vi "ME_acquire_15_DeltaForce_Daq_steppingMode.vi"() -> ()   [LabVIEW 2015]
doc: "Use this template to build a producer/consumer design pattern. Use this template when you need to execute a process, such as data analysis, when a data source, such as a triggered acquisition, produces data at an uneven rate and you need to execute the process when the data becomes available."
uses:
  oxford_driver/Oxford Drivers/BUSGEN.LLB/OxfordAddress.ctl
  <vilib>/express/express arith-compare/Formula/XNode/ExpressFormulaBlockNode.xnode
  Mode.ctl
  <vilib>/Utility/file.llb/Write Delimited Spreadsheet (DBL).vi
  <vilib>/Analysis/NI_AALBase.lvlib
  <vilib>/Analysis/baseanly.llb/Mean (DBL).vi
  <vilib>/DAQmx/configure/timing.llb/DAQmx Timing (Sample Clock).vi
  <vilib>/DAQmx/create/channels.llb/DAQmx Create Channel (AI-Voltage-Basic).vi
  <vilib>/DAQmx/read.llb/DAQmx Read (Analog 1D DBL 1Chan NSamp).vi
panel:
  out "remaining elements 2":T1(array[cluster])
  out "Actual mean":dbl format="%0.6f"
  in  "Averaged dt":dbl[][](array[numeric])
  in  "Averaged P(B)":dbl[][](array[numeric])
  out "LockInR":dbl
  out "deltaUaux":dbl
  out "Actual Voltage (V)":dbl caption="Actual AuxV" step=0.1
  in  "Stop":bool
  out "SaveSweep":bool=TRUE
  out "Measurement File_dn":path
  out "Measurement File_up":path
  out "Measurement File_average":path
  out "Actual Polarization":dbl
  in  "Reset IB?":bool
  in  "First?":bool
  in  "Save Period":dbl=1.0
  out "Averaged I(B)":dbl[][](array[numeric])
  out "P(uC/mm^2)":dbl[](array[numeric])
  in  "Sweep":bool
  out "Offset array":dbl[](array[numeric])
  in  "stop 2":bool
  in  "dB":dbl=0.005
  in  "Dwell Time (ms)":u32=1
  out "appended array":dbl[][](array[numeric])
  out "Actual B Field (T)":dbl
  out "Actual Temperature (K)":dbl
  out "Actual Current (pA)":dbl
  in  "Tab Control":T2(tab)
  in  "Max temperature (K)":dbl=20.0
  in  "Min Temperature (K)":dbl=4.5
  out "P(T)":cluster{"yi":dbl[], dbl[]}(graph)
  out "I(T)":cluster{dbl[], dbl[]}(graph)
  in  "Set temperature (K)":dbl=4.5
  in  "Temp Ramping Rate (K/min)":dbl=10.0
  in  "Heater Range":enum16{"Off", "Low", "Medium", "High"}(ring)
  in  "Heater On/Off":bool
  out "Setpoint Temperature (K)":dbl
  in  "StepField":bool
  out "I(B) 3":cluster{dbl[], dbl[]}[](graph)
  out "I(B) /Averaged/":cluster{"B array":dbl[], dbl[]}[](graph)
  out "P(B) /Averaged/":cluster{"B array":dbl[], dbl[]}[](graph)
  out "P(B)":cluster{"yi":dbl[], dbl[]}(graph)
  in  "Set Field (T)":dbl
  in  "Go to Set":bool
  in  "Sweep Rate (T/min)":dbl=2.0 format="%.6f"
  in  "Field To Zero":bool
  out "Target Field":dbl
  in  "Min Field (T)":dbl
  in  "Max Field (T)":dbl=0.15
  in  "Threshold B (T)":dbl
  out "Up/Down":bool
  in  "Dwell Time (s)":dbl=0.1
  in  "Max count array":i32[](array[numeric])=[2, 1, 0, 0, 0, 9, 10, 11, 12]
  in  "secs to wait":dbl=180.0
  out "Wait (s)":dbl
  in  "Directory":string
  out "Finished":bool=TRUE
  out "Step Rate":bool
  out "New":bool=TRUE
  in  "Temperature Array":dbl[](array[numeric])=[4.5, 5.0, 6.0, 7.0, 8.0, 9.0, 10.0, 11.0, 12.0]
  in  "Sweep Rate Array":dbl[](array[numeric])=[2.0, 1.0, 0.5, 0.1, 0.05, 9.0, 10.0, 11.0, 12.0]
  in  "Record ALL":bool
  in  "Max Countl":i32
  out "i":i32
  out "j":i32
  out "Step Temp":bool
  in  "FileName":string
  in  "Measure Noise":bool
  in  "Cycles":i32
  in  "maximum value":dbl=10.0 format="%0.2f"
  in  "minimum value":dbl=-10.0 format="%0.2f"
  in  "physical channels":tag="Dev1/ai1"
  out "PSD (pA/Hz^1/2) Peaks Removed":cluster{"f0":dbl, "df":dbl, "magnitude":dbl[]}(graph)
  out "PSD (pA/Hz^1/2)":cluster{"f0":dbl, "df":dbl, "magnitude":dbl[]}(graph)
  out "Current (pA) Filtered":waveform(dbl)(graph)
  out "Current (pA)":dbl[](graph)
  in  "Samples per channel":i32=1000
  in  "Rate":dbl=1000.0 format="%0.2f"
  in  "Cut-Off Frequency":dbl=100.0 caption="Lower Cut-Off"
  in  "Filter On":bool
  in  "First offset?":bool
  in  "Lock_in_Amplifier":refnum<visa-resource-name>="GPIB0::5::INSTR"
  out "Dc offset":dbl
  in  "Calibrate":bool
  in  "IV converter":refnum<visa-resource-name>="GPIB0::20::INSTR"
  in  "Magnetic Field":refnum<visa-resource-name>="GPIB0::21::INSTR"
  out "Time Lag":dbl=0.0500025749206543
  in  "Lake Shore":refnum<visa-resource-name>="GPIB0::11::INSTR"
  in  "Temp Refresh (s)":dbl=0.1
  in  "Sampling rate (Hz)":dbl=10.0
  in  "Gain (V/A)":dbl=1000000000.0
  in  "Sample area (mm^2)":dbl=3.9
  out "B_V":cluster{dbl[], "Best Linear Fit":dbl[]}[](graph)=[{[-0.00854253601, 0.00626134724, 0.0219834428, 0.0379117736, 0.0535871506, 0.0694316728, 0.0851615152, 0.100816481, 0.116478038, 0.132148461, 0.147876163, 0.16341701, 0.178976744, 0.194563632, 0.210251739, 0.225738944, 0.241298253, 0.256806034, 0.272344374, 0.287933477, 0.303494709, 0.318997125, 0.334591297, 0.350146681, 0.365618053, 0.380940961, 0.39666457, 0.412213675, 0.427724671, 0.443221444, 0.458760641, 0.474360042, 0.489915118, 0.505330598, 0.520967119, 0.536347531, 0.551813711, 0.567441155, 0.582995861, 0.598507522, 0.614041988, 0.629563151, 0.645106262, 0.660611914, 0.676136149, 0.691553948, 0.7071244, 0.72262999, 0.738171137, 0.753700392, 0.76919513, 0.784778028, 0.800215944, 0.8156961, 0.831325434, 0.846852183, 0.862326812, 0.877819169, 0.893312568, 0.90888536, 0.924354789], "Best Linear Fit"=[0.0, 0.005, 0.01, 0.015, 0.02, 0.025, 0.03, 0.035, 0.04, 0.045, 0.05, 0.055, 0.06, 0.065, 0.07, 0.075, 0.08, 0.085, 0.09, 0.095, 0.1, 0.105, 0.11, 0.115, 0.12, 0.125, 0.13, 0.135, 0.14, 0.145, 0.15, 0.155, 0.16, 0.165, 0.17, 0.175, 0.18, 0.185, 0.19, 0.195, 0.2, 0.205, 0.21, 0.215, 0.22, 0.225, 0.23, 0.235, 0.24, 0.245, 0.25, 0.255, 0.26, 0.265, 0.27, 0.275, 0.28, 0.285, 0.29, 0.295, 0.3]}, {[-0.00854253601, 0.00626134724, 0.0219834428, 0.0379117736, 0.0535871506, 0.0694316728, 0.0851615152, 0.100816481, 0.116478038, 0.132148461, 0.147876163, 0.16341701, 0.178976744, 0.194563632, 0.210251739, 0.225738944, 0.241298253, 0.256806034, 0.272344374, 0.287933477, 0.303494709, 0.318997125, 0.334591297, 0.350146681, 0.365618053, 0.380940961, 0.39666457, 0.412213675, 0.427724671, 0.443221444, 0.458760641, 0.474360042, 0.489915118, 0.505330598, 0.520967119, 0.536347531, 0.551813711, 0.567441155, 0.582995861, 0.598507522, 0.614041988, 0.629563151, 0.645106262, 0.660611914, 0.676136149, 0.691553948, 0.7071244, 0.72262999, 0.738171137, 0.753700392, 0.76919513, 0.784778028, 0.800215944, 0.8156961, 0.831325434, 0.846852183, 0.862326812, 0.877819169, 0.893312568, 0.90888536, 0.924354789], "Best Linear Fit"=[-0.00022554388023060128, 0.004536267537808887, 0.009593430775915074, 0.014716931562355689, 0.01975906732634002, 0.024855610270593523, 0.029915265354287977, 0.03495083565949541, 0.03998852608757118, 0.045029068349812316, 0.05008803495326229, 0.055086897848955874, 0.060091835929837946, 0.06510550835596321, 0.07015173884687344, 0.07513334727738563, 0.08013814865293042, 0.08512637555172443, 0.0901244320467579, 0.09513881694893507, 0.10014423687592358, 0.10513073807087174, 0.11014675346564809, 0.1151502923271957, 0.12012680792099008, 0.1250555686413888, 0.1301132186920259, 0.13511473785283767, 0.14010399888730068, 0.14508868495702945, 0.1500870171143548, 0.15510471446726903, 0.16010815425765457, 0.16506669165212906, 0.17009632901003072, 0.1750435864450521, 0.18001843198211442, 0.1850451496356715, 0.19004847041199868, 0.1950379453501071, 0.20003475573578386, 0.20502728708357412, 0.21002687821664084, 0.21501442030211, 0.220007939788244, 0.2249672231113706, 0.22997560874002893, 0.23496313088260184, 0.23996209027618054, 0.24495722449359253, 0.24994125598600042, 0.2549536449902534, 0.25991939913989753, 0.2648987401917687, 0.26992606578200207, 0.2749203939204135, 0.2798979571595809, 0.2848812227804405, 0.2898648235706211, 0.2948739618827834, 0.2998498524919418]}]
  out "V_I":cluster{dbl[], "Best Linear Fit":dbl[]}[](graph)=[{[0.0, 0.035, 0.069, 0.104, 0.138, 0.173, 0.208, 0.242, 0.277, 0.311, 0.346, 0.38, 0.415, 0.45, 0.484, 0.519, 0.553, 0.588, 0.623, 0.657, 0.692, 0.726, 0.761, 0.796, 0.83, 0.865, 0.899, 0.934, 0.969, 1.003, 1.038, 1.072, 1.107, 1.141, 1.176, 1.211, 1.245, 1.28, 1.314, 1.349, 1.384, 1.418, 1.453, 1.487, 1.522, 1.557, 1.591, 1.626, 1.66, 1.695, 1.73, 1.764, 1.799, 1.833, 1.868, 1.902, 1.937, 1.972, 2.006, 2.041, 2.075], "Best Linear Fit"=[-0.00854253601, 0.00626134724, 0.0219834428, 0.0379117736, 0.0535871506, 0.0694316728, 0.0851615152, 0.100816481, 0.116478038, 0.132148461, 0.147876163, 0.16341701, 0.178976744, 0.194563632, 0.210251739, 0.225738944, 0.241298253, 0.256806034, 0.272344374, 0.287933477, 0.303494709, 0.318997125, 0.334591297, 0.350146681, 0.365618053, 0.380940961, 0.39666457, 0.412213675, 0.427724671, 0.443221444, 0.458760641, 0.474360042, 0.489915118, 0.505330598, 0.520967119, 0.536347531, 0.551813711, 0.567441155, 0.582995861, 0.598507522, 0.614041988, 0.629563151, 0.645106262, 0.660611914, 0.676136149, 0.691553948, 0.7071244, 0.72262999, 0.738171137, 0.753700392, 0.76919513, 0.784778028, 0.800215944, 0.8156961, 0.831325434, 0.846852183, 0.862326812, 0.877819169, 0.893312568, 0.90888536, 0.924354789]}, {[0.0, 0.035, 0.069, 0.104, 0.138, 0.173, 0.208, 0.242, 0.277, 0.311, 0.346, 0.38, 0.415, 0.45, 0.484, 0.519, 0.553, 0.588, 0.623, 0.657, 0.692, 0.726, 0.761, 0.796, 0.83, 0.865, 0.899, 0.934, 0.969, 1.003, 1.038, 1.072, 1.107, 1.141, 1.176, 1.211, 1.245, 1.28, 1.314, 1.349, 1.384, 1.418, 1.453, 1.487, 1.522, 1.557, 1.591, 1.626, 1.66, 1.695, 1.73, 1.764, 1.799, 1.833, 1.868, 1.902, 1.937, 1.972, 2.006, 2.041, 2.075], "Best Linear Fit"=[-0.007846580254753975, 0.007882153481927697, 0.02316149482613275, 0.03889022856281441, 0.054169569907019474, 0.06989830364370113, 0.08562703738038281, 0.10090637872458785, 0.11663511246126955, 0.1319144538054746, 0.14764318754215625, 0.1629225288863613, 0.17865126262304296, 0.19437999635972467, 0.2096593377039297, 0.22538807144061138, 0.24066741278481643, 0.25639614652149806, 0.27212488025817977, 0.2874042216023848, 0.3031329553390665, 0.31841229668327153, 0.3341410304199532, 0.3498697641566349, 0.3651491055008399, 0.3808778392375216, 0.39615718058172666, 0.4118859143184083, 0.42761464805509, 0.442893989399295, 0.45862272313597674, 0.4739020644801818, 0.48963079821686345, 0.5049101395610684, 0.5206388732977502, 0.5363676070344319, 0.5516469483786369, 0.5673756821153185, 0.5826550234595236, 0.5983837571962053, 0.6141124909328869, 0.629391832277092, 0.6451205660137737, 0.6603999073579787, 0.6761286410946604, 0.691857374831342, 0.7071367161755471, 0.7228654499122288, 0.7381447912564338, 0.7538735249931156, 0.7696022587297972, 0.7848816000740022, 0.8006103338106839, 0.815889675154889, 0.8316184088915707, 0.8468977502357756, 0.8626264839724573, 0.878355217709139, 0.893634559053344, 0.9093632927900257, 0.9246426341342309]}]
  out "B0 (T)":dbl=0.0025222449819540214
  out "B/V (T/V)":dbl=0.321659617116981
  out "I0 (A)":dbl=-0.007846580254753975
  out "V/I (Ohm)":dbl=0.44939239247661916
  in  "Offset?":bool
  in  "Magnet":bool
  in  "Ramp":bool=TRUE
  in  "DaQ":bool
  in  "Moving average":i8=10
  in  "Sample Rate":dbl=1000.0
  in  "Number of Samples":i32=100
  in  "Physical Channel":tag="kartya/ai0"
  in  "Min Voltage":dbl=-5.0
  in  "Max Voltage":dbl=5.0
  in  "Terminal Configuration":i32(ring)=-1 items=["default"=-1, "RSE"=10083, "NRSE"=10078, "Differential"=10106, "Pseudodifferential"=12529]
  in  "Count":i32=100
  in  "Temp/Magnetic Field":bool
  out "index":i8
  out "Read?":bool
  out "Magnetic Field (T)":dbl[](array[numeric])
  out "Reset":bool
  out "Measured Current (pA)":dbl[](array[numeric])
  out "Elapsed Time (s)":dbl[](array[numeric])
  out "Start time":timestamp
  in  "Enum":T3=enum."Process"
  out "B array":dbl[](array[numeric])
  in  "dB (T)":dbl=0.0025
  in  "Counter":i8
  out "L magnet (H)":dbl
  out "R magnet (mOhm)":dbl
  out "Actual Current (R0)":dbl
  out "Actual Field (T)":dbl
  out "Temperature array":dbl[](array[numeric])
  in  "New Measurement File":bool
  out "Measurement File":path
  out "refnum out":refnum<file>
  in  "Measuring":bool
  in  "Measure /Pause":bool
  in  "stop":bool
  # "DeltaForce"
  # "Discrete"
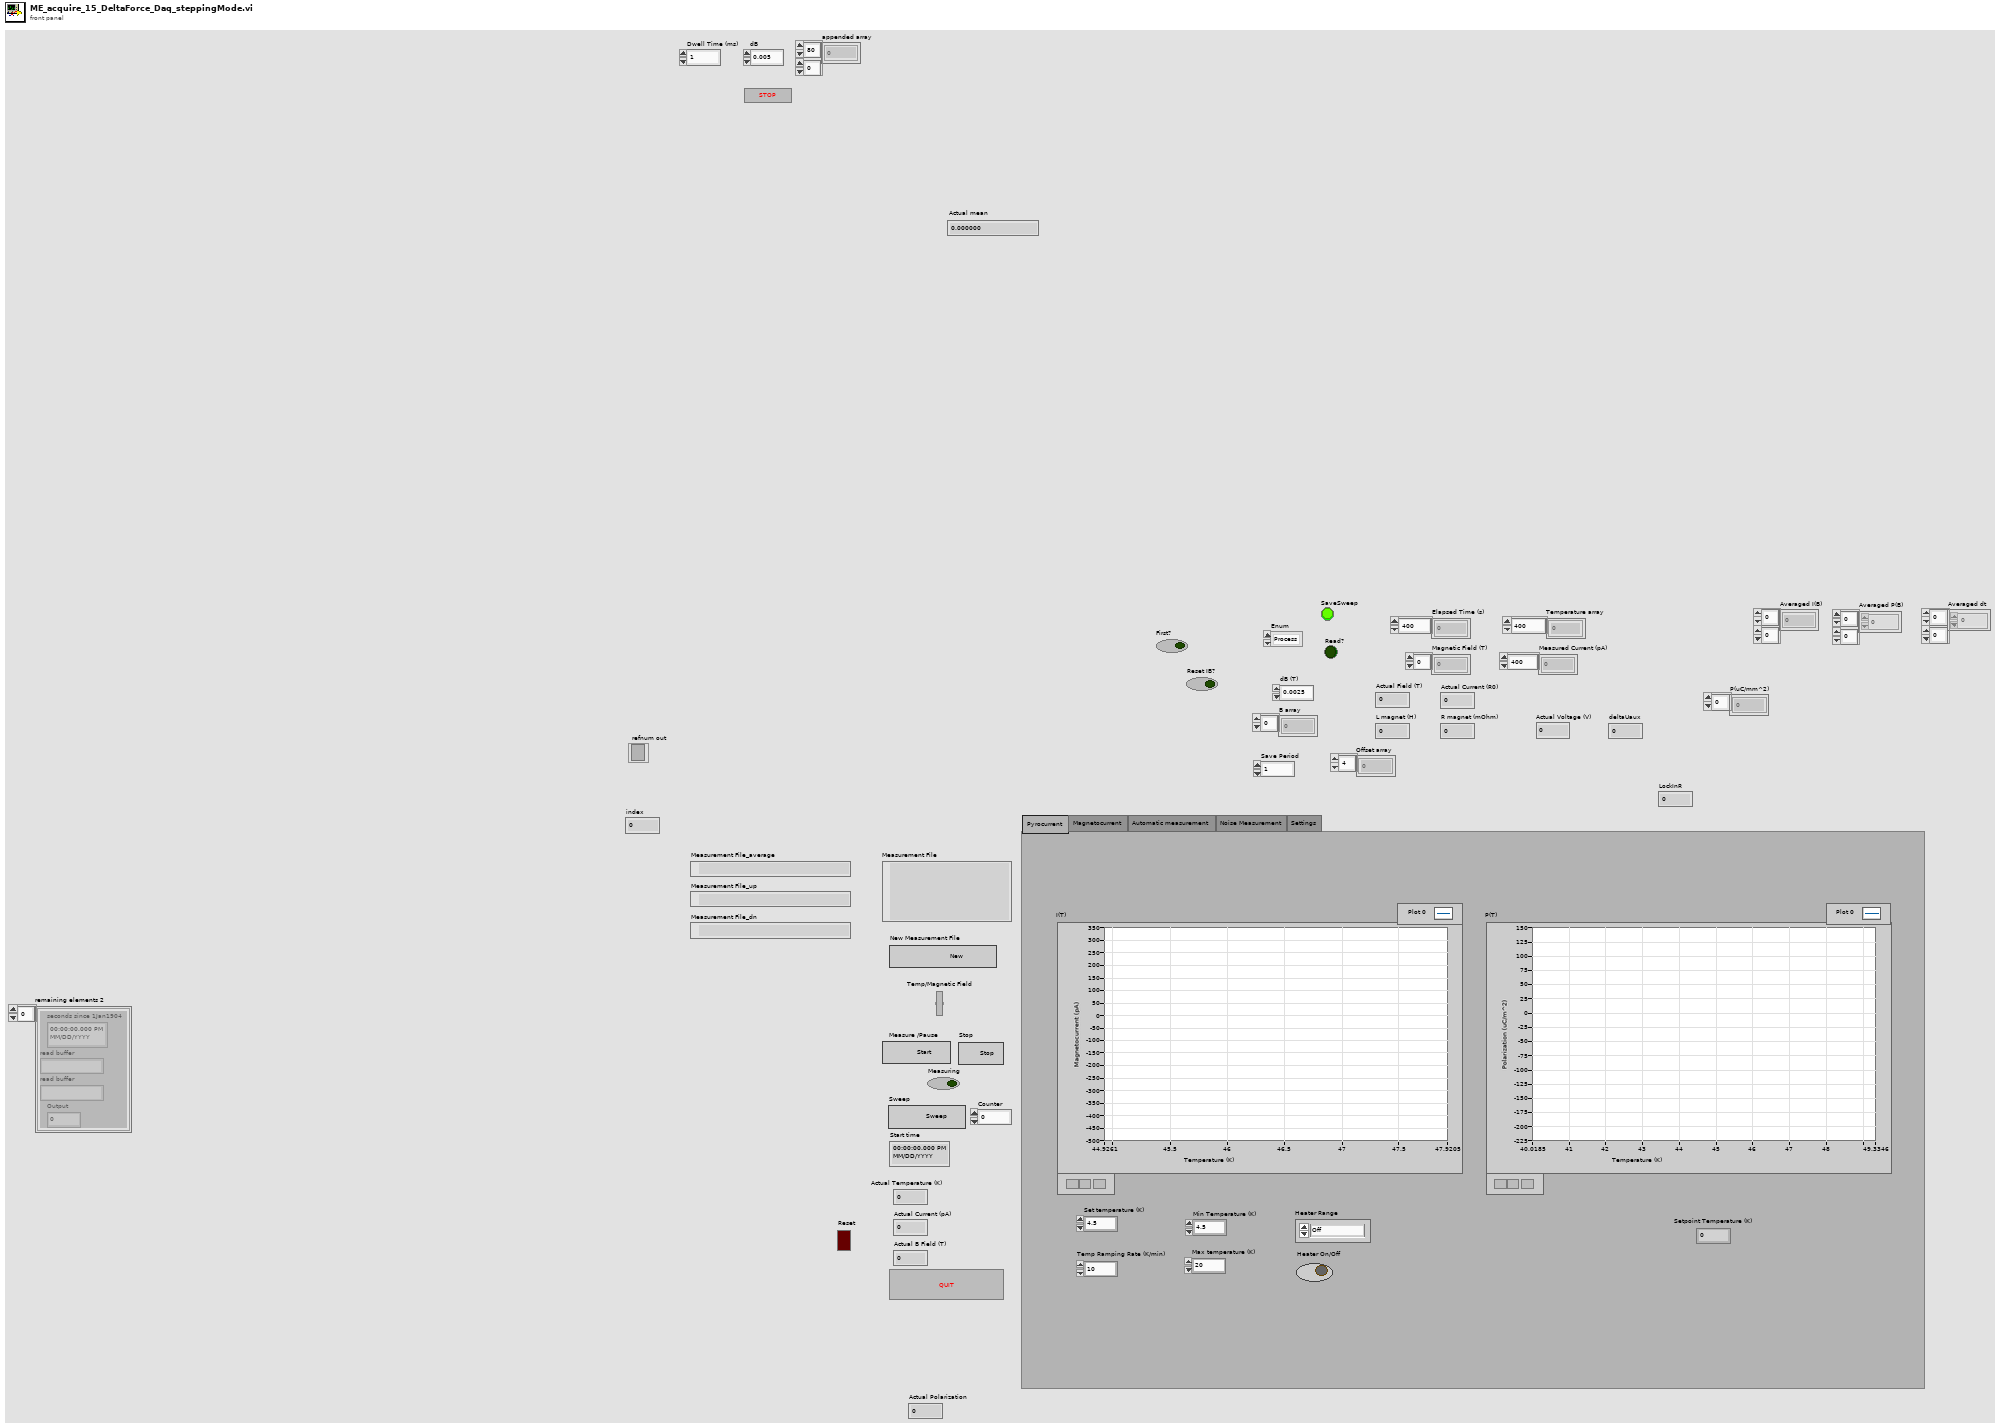
[diagram p1: front panel]
types:
  T1 = cluster{"seconds since 1Jan1904":timestamp, "read buffer":string, "read buffer":string, "Output":dbl}[]
  T2 = enum32{"Pyrocurrent", "Magnetocurrent", "Automatic measurement", "Noise Measurement", "Settings"}
  T3 = typedef "Mode.ctl" = enum16{"Offset", "Process", "Sweep", "StepOxford", "StepDelta", "Plot", "Save", "New", "Return", ""}
  T4 = cluster{"seconds since 1Jan1904":timestamp, "read buffer":string, "read buffer":string, "Output":dbl}
  T5 = enum16{"open", "replace", "create", "open or create", "replace or create", "replace or create with confirmation"}
  T6 = typedef "OxfordAddress.ctl" = cluster{"Com Port":i32, "ISOBUS Address":i32, "GPIB Address":i16, "Communication":enum16{"RS232", "ISOBUS", "GPIB", "Gateway"}}
  T7 = cluster{"B array":dbl[], "Averaged P(B) Out":dbl[]}
  T8 = cluster{"B array":dbl[], "BaselineSubtracted I(B)":dbl[]}
  T9 = cluster{"B array":dbl[], "Averaged P(B) Out":dbl[]}[]
  T10 = cluster{"B array":dbl[], "BaselineSubtracted I(B)":dbl[]}[]
  T11 = cluster{"I array out (A)":dbl[], "V array out (V)":dbl[]}
  T12 = cluster{"I array out (A)":dbl[], "Best Linear Fit":dbl[]}
  T13 = cluster{"V array out (V)":dbl[], "B array Out":dbl[]}
  T14 = cluster{"V array out (V)":dbl[], "Best Linear Fit 2":dbl[]}
  T15 = cluster{"I array out (A)":dbl[], "Best Linear Fit":dbl[]}[]
  T16 = cluster{"V array out (V)":dbl[], "Best Linear Fit 2":dbl[]}[]
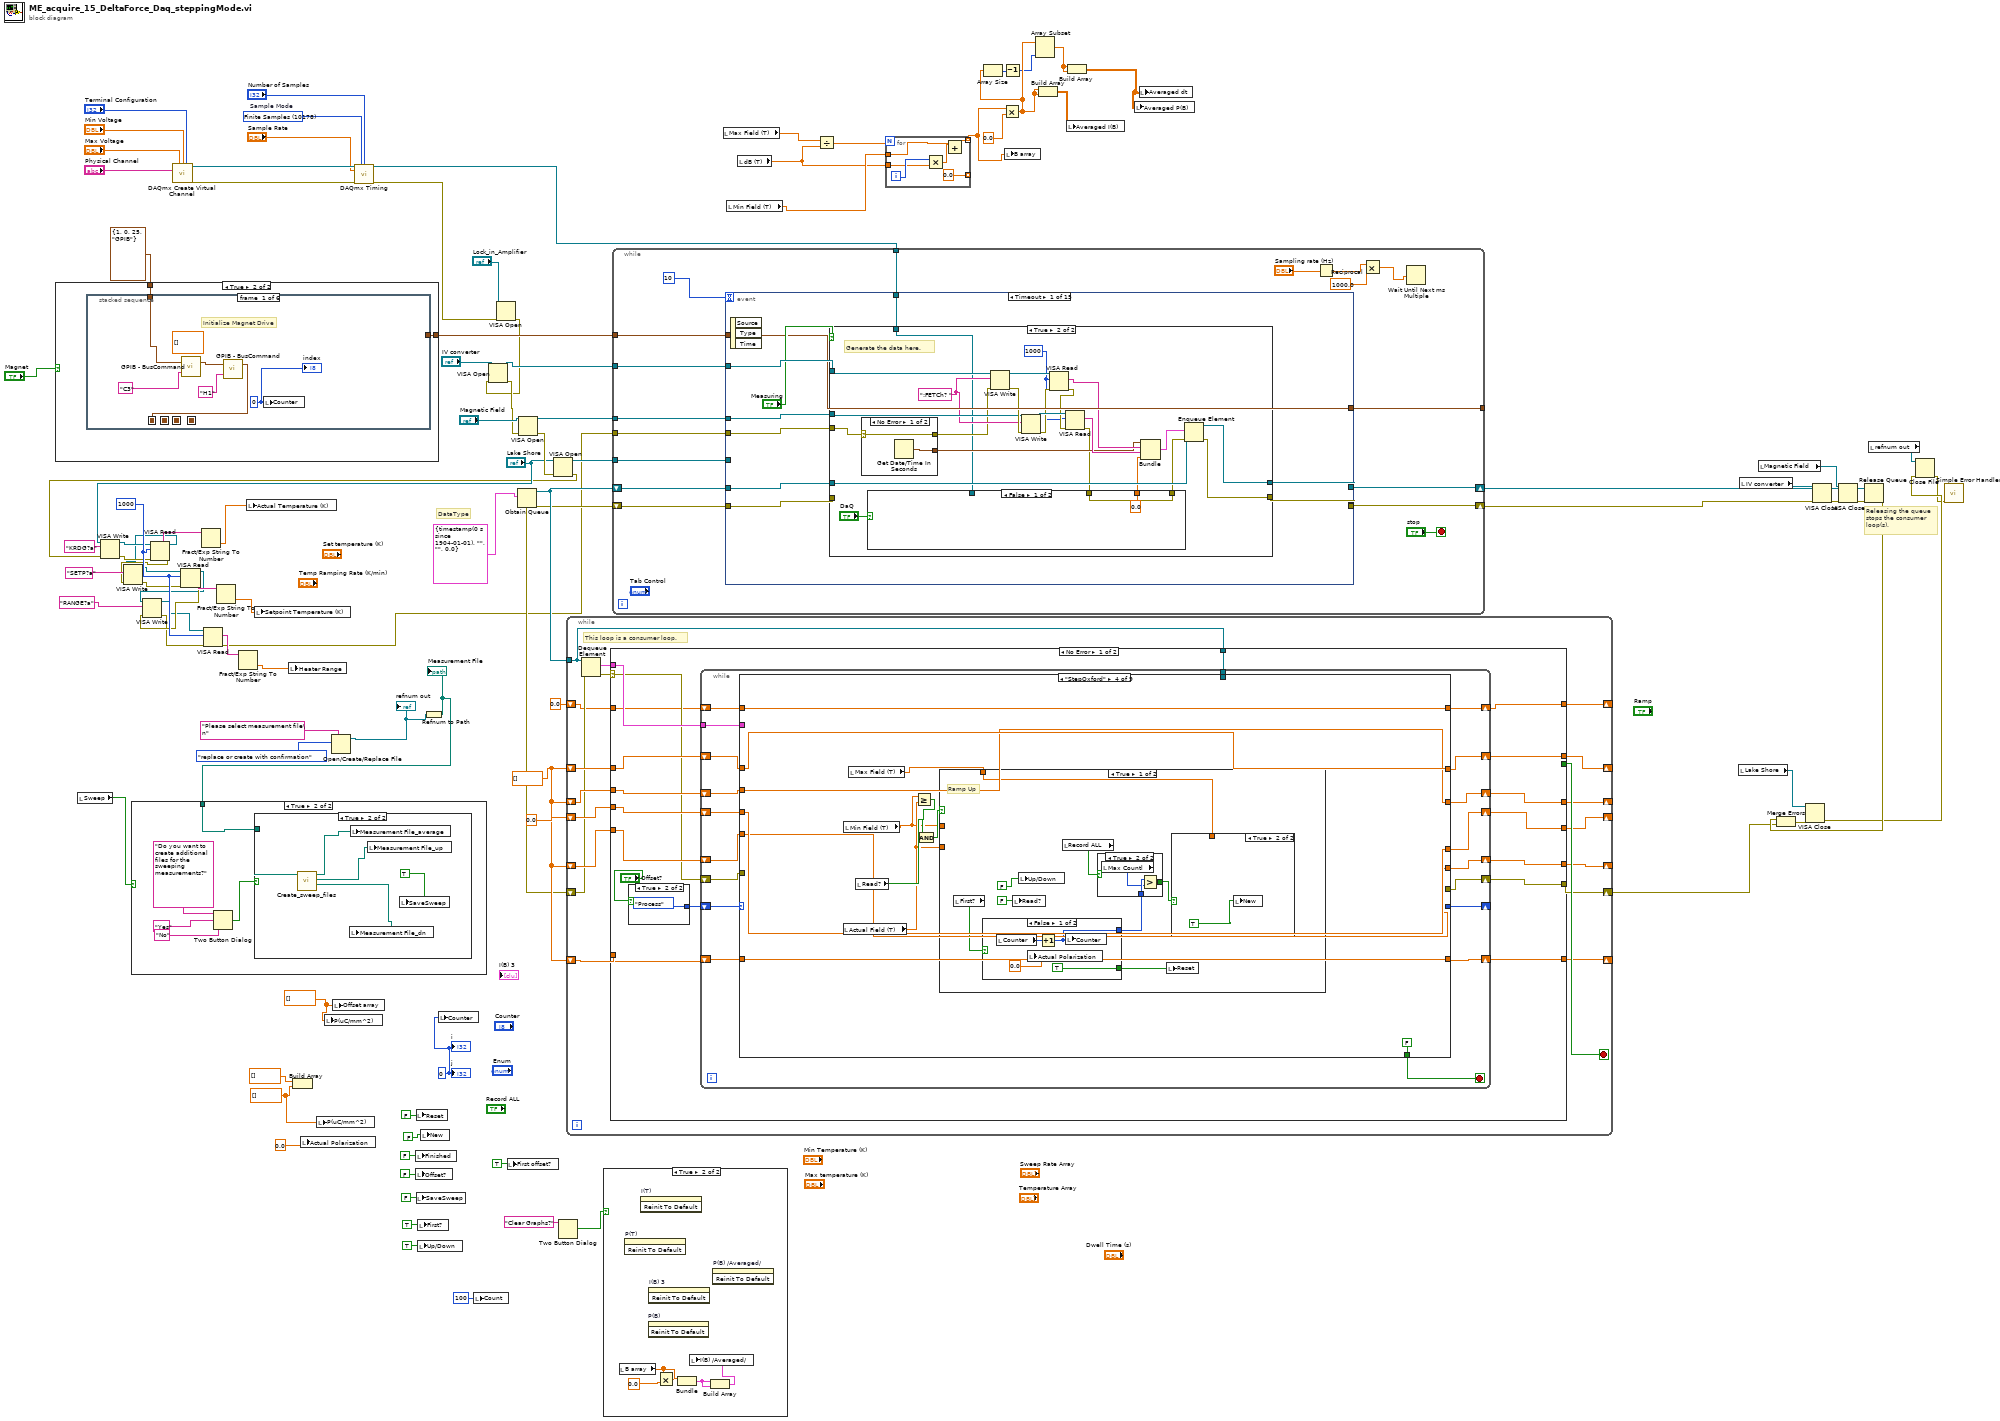
[diagram p0: block diagram]
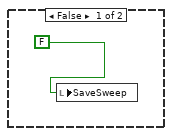
[diagram p4: hidden frame]
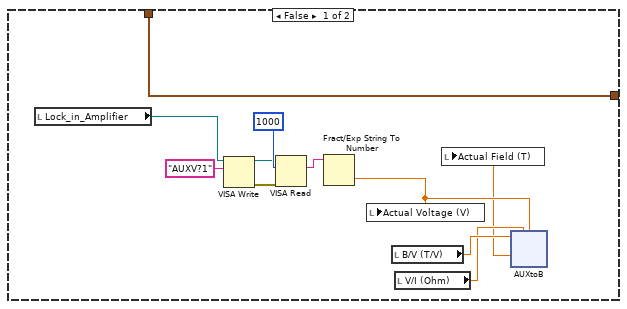
[diagram p5: hidden frame]
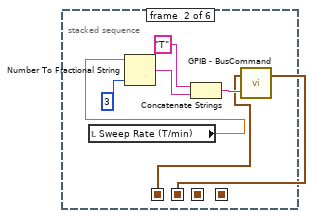
[diagram p6: hidden frame]
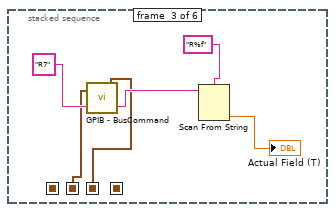
[diagram p7: hidden frame]
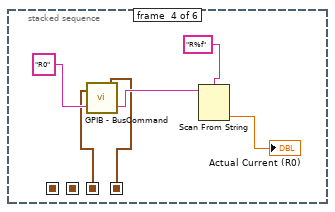
[diagram p8: hidden frame]
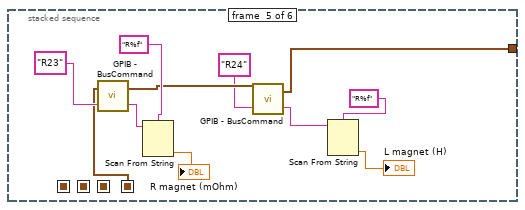
[diagram p9: hidden frame]
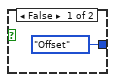
[diagram p11: hidden frame]
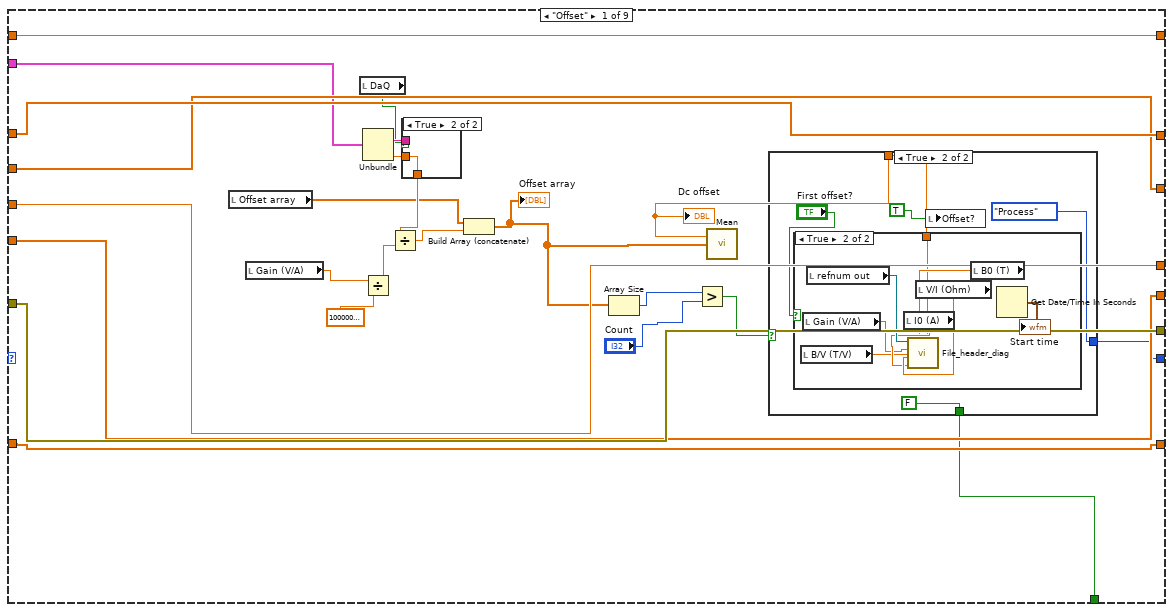
[diagram p12: hidden frame]
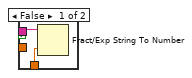
[diagram p13: hidden frame]
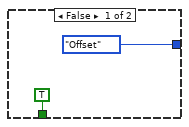
[diagram p14: hidden frame]
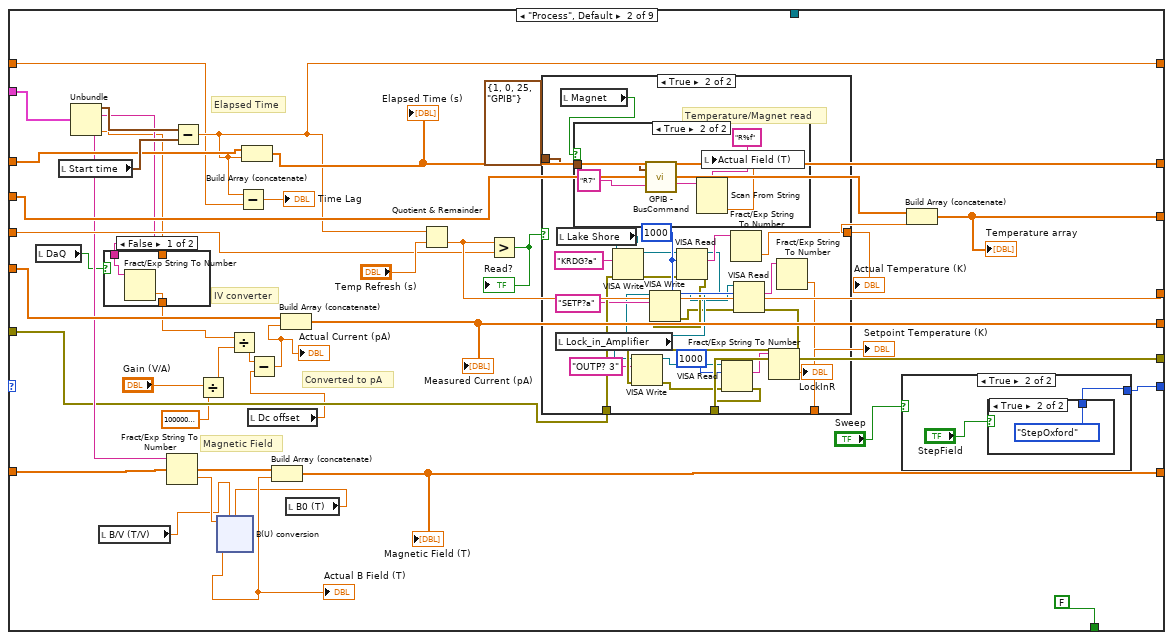
[diagram p16: hidden frame]
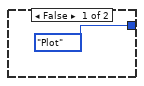
[diagram p18: hidden frame]
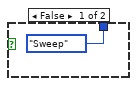
[diagram p19: hidden frame]
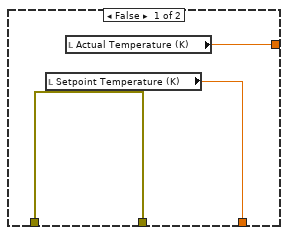
[diagram p20: hidden frame]
diagram:
  w14 = 10178 items=["Finite Samples"=10178, "Continuous Samples"=10123, "Hardware Timed Single Point"=12522]  # Sample Mode
  w41 = u32 1000 ("byte count")
  w52 = 0 ("j")
  w49 = dbl[] []
  w67 = dbl[] []
  w73 = dbl[] []
  # "DataType"
  # "Releasing the queue stops the consumer loop(s)."
  n1 = case shown="True" "Magnet" {
    tunnel: T6 {"Com Port"=1, "ISOBUS Address"=0, "GPIB Address"=25, "Communication"=enum."GPIB"} ("Address") -> [w109 w123]
    tunnel: [w109 w122] -> w79
    frame False {
      n2 = local read "Lock_in_Amplifier"() -> (w103:refnum<visa-resource-name>)
      n3 = VISA Write(VISA resource name=w103, write buffer="AUXV?1") -> (VISA resource name out=w104:refnum<visa-resource-name>, error out=w108:errorcluster)  [unwired: 1 in, 1 out]
      n4 = VISA Read(VISA resource name=w104, byte count=u32 1000, error in (no error)=w108) -> (read buffer=w107:string)  [unwired: 3 out]
      n5 = Fract/Exp String To Number(string=w107) -> (number=w100:dbl)  [unwired: 3 in, 1 out]
      n6 = local write "Actual Voltage (V)"(w100) -> ()
      n7 = local read "B/V (T/V)"() -> (w102:dbl)
      n8 = local read "V/I (Ohm)"() -> (w101:dbl)
      n9 = xnode "AUXtoB"("BpV"=w102, "Rm"=w101, "Aux"=w100) -> ("Result"=w99:dbl)  [unwired: 1 in, 1 out]
      n10 = local write "Actual Field (T)"(w99) -> ()
    }
    frame True {
      n11 = stacked-sequence {
        seq-local: [w126 _ _ _ _ _] -> [_ w131 _ _ _ _]
        seq-local: [_ w130 _ _ _ _] -> [_ _ w138 _ _ _]
        seq-local: [_ _ w137 _ _ _] -> [_ _ _ w144 _ _]
        seq-local: [_ _ _ w143 _ _] -> [_ _ _ _ w155 _]
        tunnel: w123 -> [w128 _ _ _ _ _]
        tunnel: [_ _ _ _ w153 _] -> w122
        frame #0 {
          (unwired) dbl[][] []
          w124 = i8 0 ("Counter")
          # "Initialize Magnet Drive"
          n12 = call "GPIB - BusCommand.vi"("Command"="C3", "Address"=w128) -> ("Address(thru)"=w127:T6)  [unwired: 1 out]
          n13 = call "GPIB - BusCommand.vi"("Command"="H1", "Address"=w127) -> ("Address(thru)"=w126:T6)  [unwired: 1 out]
          n14 = local write "Counter"(w124) -> ()
          "index" <- w124
        }
        frame #1 {
          n15 = local read "Sweep Rate (T/min)"() -> (w132:dbl)
          n16 = Number To Fractional String(number=w132, precision (6)=i16 3) -> (F-format string=w134:string)  [unwired: 2 in]
          n17 = Concatenate Strings("T" ("format string"), w134) -> (w133:string)
          n18 = call "GPIB - BusCommand.vi"("Command"=w133, "Address"=w131) -> ("Address(thru)"=w130:T6)  [unwired: 1 out]
        }
        frame #2 {
          n19 = call "GPIB - BusCommand.vi"("Command"="R7" ("format string"), "Address"=w138) -> ("Reply"=w142:string, "Address(thru)"=w137:T6)
          n20 = Scan From String(format string="R%f" ("remaining string"), input string=w142) -> (output 1=→"Actual Field (T)":dbl)  [unwired: 3 in, 3 out]
        }
        frame #3 {
          n21 = call "GPIB - BusCommand.vi"("Command"="R0" ("format string"), "Address"=w144) -> ("Reply"=w148:string, "Address(thru)"=w143:T6)
          n22 = Scan From String(format string="R%f" ("remaining string"), input string=w148) -> (output 1=→"Actual Current (R0)":dbl)  [unwired: 3 in, 3 out]
        }
        frame #4 {
          n23 = call "GPIB - BusCommand.vi"("Command"="R23" ("format string"), "Address"=w155) -> ("Reply"=w159:string, "Address(thru)"=w154:T6)
          n24 = Scan From String(format string="R%f" ("remaining string"), input string=w159) -> (output 1=→"R magnet (mOhm)":dbl)  [unwired: 3 in, 3 out]
          n25 = call "GPIB - BusCommand.vi"("Command"="R24" ("format string"), "Address"=w154) -> ("Reply"=w151:string, "Address(thru)"=w153:T6)
          n26 = Scan From String(format string="R%f" ("remaining string"), input string=w151) -> (output 1=→"L magnet (H)":dbl)  [unwired: 3 in, 3 out]
        }
        frame #5 {
        }
      }
    }
  }
  n27 = local read "Sweep"() -> (w57:bool)
  n28 = call-poly <vilib>:"DAQmx Create Virtual Channel.vi"("maximum value"="Max Voltage", "minimum value"="Min Voltage", "input terminal configuration"="Terminal Configuration", "physical channels"="Physical Channel") -> ("task out"=w12:refnum<k21>, "error out"=w13:errorcluster)  [unwired: 10 in]
  n29 = Build Array(dbl[] [], w49) -> ()  [unwired: 1 out]
  n30 = local write "Actual Polarization"(0.0 ("Actual Polarization")) -> ()
  n31 = local write "P(uC/mm^2)"(w49) -> ()
  n32 = local write "P(uC/mm^2)"(w67) -> ()
  n33 = Open/Create/Replace File(prompt="Please select measurement file\n", operation (0:open)=T5."replace or create with confirmation") -> (refnum out=w76:refnum<file>)  [unwired: 4 in, 2 out]
  "refnum out" <- w76
  n34 = local write "Offset array"(w67) -> ()
  n35 = call-poly <vilib>:"DAQmx Timing.vi"("task/channels in"=w12, "sample mode"=w14, "samples per channel"="Number of Samples", "rate"="Sample Rate", "error in"=w13) -> ("task out"=w4:refnum<k21>, "error out"=w5:errorcluster)  [unwired: 9 in]
  n36 = local write "Finished"(FALSE ("Finished")) -> ()
  n37 = local write "Offset?"(FALSE ("Offset?")) -> ()
  n38 = local write "Reset"(FALSE ("Reset")) -> ()
  n39 = local write "SaveSweep"(FALSE ("SaveSweep")) -> ()
  n40 = local write "First?"(TRUE ("First?")) -> ()
  n41 = local write "Up/Down"(TRUE ("Up/Down")) -> ()
  n42 = local write "New"(FALSE ("New")) -> ()
  n43 = Refnum to Path(1:w76) -> (0:w56:path)
  "Measurement File" <- w56
  n44 = case shown="True" w57 {
    tunnel: w56 -> [_ w160]
    frame False {
    }
    frame True {
      n45 = Two Button Dialog(message="Do you want to create additional files for the sweeping measurements?" ("string"), 1:"No" ("F button name (\"Cancel\")"), 2:"Yes" ("T button name (\"OK\")")) -> (T button?=w162:bool)
      n46 = case shown="True" w162 {
        tunnel: w160 -> [_ w170]
        frame False {
          n47 = local write "SaveSweep"(FALSE ("SaveSweep")) -> ()
        }
        frame True {
          n48 = call "Create_sweep_files.vi"("Measurement File"=w170) -> ("Path 3"=w167:path, "Path 2"=w168:path, "Path"=w169:path)  [unwired: 8 in]
          n49 = local write "Measurement File_dn"(w167) -> ()
          n50 = local write "Measurement File_average"(w169) -> ()
          n51 = local write "Measurement File_up"(w168) -> ()
          n52 = local write "SaveSweep"(TRUE) -> ()
        }
      }
    }
  }
  n53 = local write "Counter"(w52) -> ()
  n54 = local write "Count"(100 ("Count")) -> ()
  n55 = VISA Open(error in (no error)=w5, VISA resource name="Lock_in_Amplifier") -> (error out=w24:errorcluster)  [unwired: 3 in, 1 out]
  n56 = VISA Open(error in (no error)=w24, VISA resource name="IV converter") -> (VISA resource name=w93:refnum<visa-resource-name>, error out=w95:errorcluster)  [unwired: 3 in]
  n57 = local write "First offset?"(TRUE ("First offset?")) -> ()
  n58 = Obtain Queue(element data type=T4 {"seconds since 1Jan1904"=timestamp(0 s since 1904-01-01), "read buffer"="", "read buffer"="", "Output"=0.0} ("output cluster")) -> (queue out=w98:refnum<queue>, error out=w71:errorcluster)  [unwired: 4 in, 1 out]
  n59 = VISA Open(error in (no error)=w95, VISA resource name="Magnetic Field") -> (VISA resource name=w92:refnum<visa-resource-name>, error out=w74:errorcluster)  [unwired: 3 in]
  n60 = VISA Open(error in (no error)=w74, VISA resource name="Lake Shore") -> (VISA resource name=w69:refnum<visa-resource-name>, error out=w38:errorcluster)  [unwired: 3 in]
  n61 = VISA Write(VISA resource name="Lake Shore", write buffer="KRDG?a", error in (no error)=w38) -> (VISA resource name out=w35:refnum<visa-resource-name>, error out=w34:errorcluster)  [unwired: 1 out]
  n62 = VISA Read(VISA resource name=w35, byte count=w41, error in (no error)=w34) -> (VISA resource name out=w32:refnum<visa-resource-name>, read buffer=w46:string, error out=w33:errorcluster)  [unwired: 1 out]
  n63 = VISA Write(VISA resource name=w32, write buffer="SETP?a", error in (no error)=w33) -> (VISA resource name out=w31:refnum<visa-resource-name>, error out=w30:errorcluster)  [unwired: 1 out]
  n64 = VISA Read(VISA resource name=w31, byte count=w41, error in (no error)=w30) -> (VISA resource name out=w28:refnum<visa-resource-name>, read buffer=w45:string, error out=w29:errorcluster)  [unwired: 1 out]
  n65 = VISA Write(VISA resource name=w28, write buffer="RANGE?a", error in (no error)=w29) -> (VISA resource name out=w26:refnum<visa-resource-name>, error out=w27:errorcluster)  [unwired: 1 out]
  n66 = Fract/Exp String To Number(string=w46) -> (number=w44:dbl)  [unwired: 3 in, 1 out]
  n67 = VISA Read(VISA resource name=w26, byte count=w41, error in (no error)=w27) -> (read buffer=w40:string, error out=w37:errorcluster)  [unwired: 2 out]
  n68 = Fract/Exp String To Number(string=w45) -> (number=w43:dbl)  [unwired: 3 in, 1 out]
  n69 = Fract/Exp String To Number(string=w40) -> (number=w36:dbl)  [unwired: 3 in, 1 out]
  n70 = local write "Actual Temperature (K)"(w44) -> ()
  n71 = local write "Setpoint Temperature (K)"(w43) -> ()
  n72 = local write "Heater Range"(w36) -> ()
  n73 = Two Button Dialog(message="Clear Graphs?") -> (T button?=w51:bool)  [unwired: 2 in]
  n74 = while {
    tunnel: w98 -> [w171]
    shift-right: [w184] -> _
    shift-left: w73 -> [w183]
    shift-right: [w182] -> _
    shift-left: w73 -> [w181]
    shift-right: [w180] -> _
    shift-left: w73 -> [w179]
    shift-right: [w178] -> _
    shift-left: 0.0 -> [w177]
    shift-right: [w176] -> _
    shift-left: w73 -> [w175]
    shift-right: [w185] -> w84
    shift-left: w71 -> [w174]
    shift-right: [w173] -> _
    shift-left: 0.0 -> [w172]
    stop <- w186 stop-if-true
    # "This loop is a consumer loop."
    n75 = Dequeue Element(queue=w171, error in (no error)=w174) -> (element=w187:T4, error out=w188:errorcluster)  [unwired: 1 in, 2 out]
    n76 = case shown="No Error" w188 {
      selector: w188 -> [w194 w915]
      tunnel: w187 -> [w205 _]
      tunnel: [_ TRUE] -> w186
      tunnel: [w193 w915] -> w185
      tunnel: [w204 w914] -> w184
      tunnel: w183 -> [w203 w914]
      tunnel: [w202 w911] -> w182
      tunnel: w181 -> [w201 w911]
      tunnel: [w200 w910] -> w180
      tunnel: w179 -> [w199 w910]
      tunnel: [w198 w912] -> w178
      tunnel: w177 -> [w197 w912]
      tunnel: [w196 w913] -> w176
      tunnel: w175 -> [w195 w913]
      tunnel: [w192 w909] -> w173
      tunnel: w172 -> [w191 w909]
      tunnel: w171 -> [w189 _]
      frame No Error {
        n77 = case shown="True" "Offset?" {
          tunnel: [Mode."Offset" ("Enum") Mode."Process" ("Enum")] -> w206
          frame False {
          }
          frame True {
          }
        }
        n78 = while {
          shift-right: [w215] -> _
          shift-left: w206 -> [w227]
          tunnel: w205 -> [w226]
          shift-right: [w225] -> w204
          shift-left: w203 -> [w224]
          shift-right: [w217] -> w196
          shift-left: w195 -> [w216]
          shift-right: [w219] -> w198
          shift-left: w197 -> [w218]
          shift-right: [w223] -> w202
          shift-left: w201 -> [w222]
          shift-right: [w213] -> w193
          shift-left: w194 -> [w214]
          shift-right: [w221] -> w200
          shift-left: w199 -> [w220]
          shift-right: [w211] -> w192
          shift-left: w191 -> [w210]
          tunnel: w189 -> [w209]
          stop <- w212 stop-if-true
          n79 = case shown="\"StepOxford\"" w227 {
            selector: w227 -> [_ _ _ _ _ _ _ _ w902]
            tunnel: w226 -> [w245 w308 _ _ _ _ _ _ _]
            tunnel: [w251 w305 w369 w486 w525 w587 w660 w743 w907] -> w225
            tunnel: w224 -> [w251 w298 w369 w486 w525 w587 w656 w743 w907]
            tunnel: [w246 w304 w372 w483 w523 w589 w662 w741 w904] -> w223
            tunnel: w222 -> [w246 w303 w372 w483 w523 w589 w657 w741 w904]
            tunnel: [w247 w302 w374 w482 w521 w584 w663 w739 w901] -> w221
            tunnel: w220 -> [w247 w301 w374 w482 w521 w584 w658 w739 w901]
            tunnel: [w249 w297 w371 w484 w516 w585 w666 0.0 w905] -> w219
            tunnel: w218 -> [w249 w296 w371 w484 w516 w585 w666 _ w905]
            tunnel: [w250 w293 w370 w485 w524 w586 w661 w742 w906] -> w217
            tunnel: w216 -> [w250 w294 w370 w485 w524 w586 w659 w742 w906]
            tunnel: [w235 w291 w367 _ Mode."Plot" ("Enum") Mode."Save" ("Enum") w667 Mode."Return" ("Enum") w902] -> w215
            tunnel: w214 -> [w248 w289 w376 _ w519 w592 w665 w735 w903]
            tunnel: [w248 w288 w375 _ w518 w592 w665 w734 w903] -> w213
            tunnel: [w231 FALSE FALSE FALSE FALSE FALSE w654 TRUE TRUE] -> w212
            tunnel: [w234 w285 w368 w487 w517 w588 w664 0.0 w908] -> w211
            tunnel: w210 -> [w234 w284 w368 w487 w517 w588 w664 _ w908]
            tunnel: w209 -> [_ _ _ _ _ _ _ w733 _]
            frame "Offset" {
              n80 = local read "Offset array"() -> (w239:dbl[])
              n81 = local read "Gain (V/A)"() -> (w243:dbl)
              n82 = local read "DaQ"() -> (w230:bool)
              n83 = Unbundle(w245) -> ("read buffer"=w233:string, "Output"=w229:dbl)  [unwired: 2 out]
              n84 = Divide(x=w243, y=1000000000000.0) -> (x/y=w241:dbl)
              n85 = case shown="True" w230 {
                tunnel: [w253 w254] -> w244
                tunnel: w233 -> [w252 _]
                tunnel: w229 -> [_ w254]
                frame False {
                  n86 = Fract/Exp String To Number(string=w252) -> (number=w253:dbl)  [unwired: 3 in, 1 out]
                }
                frame True {
                }
              }
              n87 = Divide(x=w244, y=w241) -> (x/y=w240:dbl)
              n88 = Build Array (concatenate)(w239, w240) -> (w236:dbl[])
              "Offset array" <- w236
              n89 = Array Size(array=w236) -> (size(s)=w238:i32)
              n90 = Greater?(x=w238, y="Count") -> (0:w237:bool)
              n91 = call-poly <vilib>:"Mean.vi"("X"=w236) -> ("mean"=w232:dbl)  [unwired: 1 out]
              "Dc offset" <- w232
              n92 = case shown="True" w237 {
                tunnel: [Mode."Offset" ("Enum") Mode."Process" ("Enum")] -> w235
                tunnel: w232 -> [_ w261]
                tunnel: [TRUE FALSE] -> w231
                frame False {
                }
                frame True {
                  n93 = case shown="True" "First offset?" {
                    tunnel: w261 -> [_ w263]
                    frame False {
                    }
                    frame True {
                      n94 = local read "B/V (T/V)"() -> (w264:dbl)
                      n95 = local read "Gain (V/A)"() -> (w265:dbl)
                      n96 = local read "refnum out"() -> (w269:refnum<file>)
                      n97 = local read "I0 (A)"() -> (w267:dbl)
                      n98 = local read "V/I (Ohm)"() -> (w268:dbl)
                      n99 = local read "B0 (T)"() -> (w266:dbl)
                      n100 = call "File_header_diag.vi"("OFFSET"=w263, "B0"=w266, "B/V"=w264, "I0"=w267, "V/I"=w268, "Gain"=w265, "Byte Stream File in"=w269) -> ()  [unwired: 5 in]
                      n101 = Get Date/Time In Seconds() -> (seconds since 1Jan1904=→"Start time":timestamp)
                    }
                  }
                  n102 = local write "Offset?"(TRUE ("Offset?")) -> ()
                }
              }
            }
            frame "Process", Default {
              # "Converted to pA"
              # "Magnetic Field"
              # "IV converter"
              # "Elapsed Time"
              n103 = local read "DaQ"() -> (w272:bool)
              n104 = local read "Start time"() -> (w306:timestamp)
              n105 = Unbundle(w308) -> ("seconds since 1Jan1904"=w307:timestamp, "read buffer"=w273:string, "read buffer"=w290:string, "Output"=w270:dbl)
              n106 = local read "B/V (T/V)"() -> (w280:dbl)
              n107 = case shown="False" w272 {
                tunnel: w273 -> [w312 _]
                tunnel: [w311 w313] -> w271
                tunnel: w270 -> [_ w313]
                frame False {
                  n108 = Fract/Exp String To Number(string=w312) -> (number=w311:dbl)  [unwired: 3 in, 1 out]
                }
                frame True {
                }
              }
              n109 = Fract/Exp String To Number(string=w290) -> (number=w300:dbl)  [unwired: 3 in, 1 out]
              n110 = Subtract(x=w307, y=w306) -> (x-y=w285:dbl)
              n111 = Divide(x="Gain (V/A)", y=1000000000000.0) -> (x/y=w283:dbl)
              n112 = Divide(x=w271, y=w283) -> (x/y=w278:dbl)
              n113 = Subtract(x=w285, y=w284) -> (x-y=→"Time Lag":dbl)
              n114 = Build Array (concatenate)(w298, w285) -> (w305:dbl[])
              "Elapsed Time (s)" <- w305
              n115 = local read "Dc offset"() -> (w276:dbl)
              n116 = Subtract(x=w278, y=w276) -> (x-y=w277:dbl)
              "Actual Current (pA)" <- w277
              n117 = Build Array (concatenate)(w303, w277) -> (w304:dbl[])
              "Measured Current (pA)" <- w304
              n118 = local read "B0 (T)"() -> (w279:dbl)
              n119 = xnode "B(U) conversion"("V"=w300, "BpV"=w280, "B0"=w279) -> ("Result"=w299:dbl)  [unwired: 1 in, 1 out]
              "Actual B Field (T)" <- w299
              n120 = Build Array (concatenate)(w301, w299) -> (w302:dbl[])
              "Magnetic Field (T)" <- w302
              n121 = Quotient & Remainder(x=w285, y="Temp Refresh (s)") -> (floor(x/y)=w297:dbl)  [unwired: 1 out]
              n122 = Greater?(x=w297, y=w296) -> (0:w295:bool)
              "Read?" <- w295
              n123 = case shown="True" w295 {
                tunnel: [w320 w345] -> w292
                tunnel: w289 -> [w321 w344]
                tunnel: [w321 w324] -> w288
                tunnel: T6 {"Com Port"=1, "ISOBUS Address"=0, "GPIB Address"=25, "Communication"=enum."GPIB"} ("Address") -> [_ w343]
                tunnel: [w319 w339] -> w274
                frame False {
                  n124 = local read "Setpoint Temperature (K)"() -> (w319:dbl)
                  n125 = local read "Actual Temperature (K)"() -> (w320:dbl)
                }
                frame True {
                  w340 = u32 1000 ("byte count")
                  # "Temperature/Magnet read"
                  n126 = local read "Lock_in_Amplifier"() -> (w328:refnum<visa-resource-name>)
                  n127 = local read "Lake Shore"() -> (w342:refnum<visa-resource-name>)
                  n128 = local read "Magnet"() -> (w331:bool)
                  n129 = case shown="True" w331 {
                    tunnel: w343 -> [_ w349]
                    frame False {
                    }
                    frame True {
                      n130 = call "GPIB - BusCommand.vi"("Command"="R7" ("format string"), "Address"=w349) -> ("Reply"=w350:string)  [unwired: 1 out]
                      n131 = Scan From String(format string="R%f" ("remaining string"), input string=w350) -> (output 1=w348:dbl)  [unwired: 3 in, 3 out]
                      n132 = local write "Actual Field (T)"(w348) -> ()
                    }
                  }
                  n133 = VISA Write(VISA resource name=w342, write buffer="KRDG?a", error in (no error)=w344) -> (VISA resource name out=w338:refnum<visa-resource-name>, error out=w336:errorcluster)  [unwired: 1 out]
                  n134 = VISA Read(VISA resource name=w338, byte count=w340, error in (no error)=w336) -> (VISA resource name out=w337:refnum<visa-resource-name>, read buffer=w346:string, error out=w335:errorcluster)  [unwired: 1 out]
                  n135 = VISA Write(VISA resource name=w337, write buffer="SETP?a", error in (no error)=w335) -> (VISA resource name out=w333:refnum<visa-resource-name>, error out=w334:errorcluster)  [unwired: 1 out]
                  n136 = Fract/Exp String To Number(string=w346) -> (number=w345:dbl)  [unwired: 3 in, 1 out]
                  n137 = VISA Read(VISA resource name=w333, byte count=w340, error in (no error)=w334) -> (read buffer=w332:string, error out=w330:errorcluster)  [unwired: 2 out]
                  n138 = VISA Write(VISA resource name=w328, write buffer="OUTP? 3", error in (no error)=w330) -> (VISA resource name out=w327:refnum<visa-resource-name>, error out=w329:errorcluster)  [unwired: 1 out]
                  n139 = VISA Read(VISA resource name=w327, byte count=u32 1000, error in (no error)=w329) -> (read buffer=w323:string, error out=w324:errorcluster)  [unwired: 2 out]
                  n140 = Fract/Exp String To Number(string=w323) -> (number=→"LockInR":dbl)  [unwired: 3 in, 1 out]
                  n141 = Fract/Exp String To Number(string=w332) -> (number=w339:dbl)  [unwired: 3 in, 1 out]
                }
              }
              "Actual Temperature (K)" <- w292
              "Setpoint Temperature (K)" <- w274
              n142 = case shown="True" "Sweep" {
                tunnel: [Mode."Plot" ("Enum") w316] -> w291
                frame False {
                }
                frame True {
                  n143 = case shown="True" "StepField" {
                    tunnel: [Mode."Sweep" ("Enum") Mode."StepOxford" ("Enum")] -> w316
                    frame False {
                    }
                    frame True {
                    }
                  }
                }
              }
              n144 = Build Array (concatenate)(w294, w292) -> (w293:dbl[])
              "Temperature array" <- w293
            }
            frame "Sweep" {
              n145 = local read "Temp/Magnetic Field"() -> (w366:bool)
              n146 = case shown="False" w366 {
                tunnel: w376 -> [w385 w442]
                tunnel: [w384 w441] -> w375
                frame False {
                  n147 = local read "Actual Field (T)"() -> (w380:dbl)
                  n148 = local read "Min Field (T)"() -> (w379:dbl)
                  n149 = local read "Max Field (T)"() -> (w386:dbl)
                  n150 = local read "Read?"() -> (w383:bool)
                  n151 = Greater Or Equal?(x=w379, y=w380) -> (x >= y?=w382:bool)
                  n152 = Compound Arithmetic op=AND(w382, w383) -> (w381:bool)
                  n153 = case shown="True" w381 {
                    tunnel: [w389 w425] -> w384
                    tunnel: w386 -> [w387 w424]
                    tunnel: w379 -> [_ w423]
                    tunnel: w380 -> [_ w421]
                    tunnel: w385 -> [w390 w420]
                    frame True {
                      # "Ramp Up"
                      n154 = case shown="False" "First?" {
                        tunnel: [TRUE ("Save") FALSE ("Save")] -> w393
                        tunnel: [w412 w416] -> w392
                        frame False {
                          n155 = local read "Counter"() -> (w415:i8)
                          n156 = local write "Actual Polarization"(0.0 ("Actual Polarization")) -> ()
                          n157 = Increment(x=w415) -> (x+1=w412:i8)
                          n158 = local write "Counter"(w412) -> ()
                        }
                        frame True {
                          n159 = local read "Counter"() -> (w416:i8)
                          n160 = local write "First?"(FALSE ("First?")) -> ()
                        }
                      }
                      "Reset" <- w393
                      n161 = local write "Read?"(FALSE ("Read?")) -> ()
                      n162 = local read "Record ALL"() -> (w388:bool)
                      n163 = case shown="True" w388 {
                        tunnel: w392 -> [_ w400]
                        tunnel: [FALSE w398] -> w391
                        frame False {
                        }
                        frame True {
                          n164 = Greater?(x=w400, y="Max Countl") -> (0:w398:bool)
                        }
                      }
                      n165 = case shown="False" w391 {
                        tunnel: w390 -> [w404 w411]
                        tunnel: [w403 w411] -> w389
                        tunnel: w387 -> [w402 _]
                        frame False {
                          n166 = local read "Magnet"() -> (w401:bool)
                          n167 = case shown="True" w401 {
                            tunnel: w404 -> [w405 w408]
                            tunnel: [w405 w407] -> w403
                            tunnel: w402 -> [_ w406]
                            frame False {
                            }
                            frame True {
                              n168 = call "Set_B.vi"("error in (no error)"=w408, "address string"="25", "Set Field (T)"=w406) -> ("error out"=w407:errorcluster)  [unwired: 8 in]
                            }
                          }
                          "Target Field" <- w402
                        }
                        frame True {
                          "New" <- TRUE
                        }
                      }
                      "Up/Down" <- FALSE ("Up/Down")
                    }
                    frame False {
                      n169 = Less Or Equal?(x=w424, y=w421) -> (x <= y?=w422:bool)
                      n170 = case shown="True" w422 {
                        tunnel: [w426 w430] -> w425
                        tunnel: w423 -> [_ w428]
                        tunnel: w420 -> [w426 w431]
                        frame False {
                        }
                        frame True {
                          # "Resetting at the end of every cycle"
                          # "Ramp Dn"
                          n171 = local write "Up/Down"(TRUE ("Up/Down")) -> ()
                          n172 = local read "Magnet"() -> (w427:bool)
                          n173 = local write "Target Field"(w428) -> ()
                          n174 = local write "Reset"(TRUE ("Reset")) -> ()
                          n175 = case shown="True" w427 {
                            tunnel: w431 -> [w433 w436]
                            tunnel: [w433 w435] -> w430
                            tunnel: w428 -> [_ w434]
                            frame False {
                            }
                            frame True {
                              n176 = call "Set_B.vi"("error in (no error)"=w436, "address string"="25", "Set Field (T)"=w434) -> ("error out"=w435:errorcluster)  [unwired: 8 in]
                            }
                          }
                        }
                      }
                      n177 = local write "Read?"(FALSE ("Read?")) -> ()
                    }
                  }
                }
                frame True {
                  n178 = local read "Setpoint Temperature (K)"() -> (w440:dbl)
                  n179 = local read "Min Temperature (K)"() -> (w439:dbl)
                  n180 = local read "Read?"() -> (w445:bool)
                  n181 = local read "Max temperature (K)"() -> (w438:dbl)
                  n182 = Equal?(x=w440, y=w439) -> (x = y?=w443:bool)
                  n183 = And(x=w443, y=w445) -> (x .and. y?=w444:bool)
                  n184 = case shown="False" w444 {
                    tunnel: [w447 w464] -> w441
                    tunnel: w438 -> [w446 w463]
                    tunnel: w439 -> [_ w462]
                    tunnel: w440 -> [_ w460]
                    tunnel: w442 -> [w448 w459]
                    frame True {
                      # "Ramp Up"
                      n185 = local read "First?"() -> (w454:bool)
                      n186 = case shown="False" w454 {
                        frame False {
                          n187 = local read "Counter"() -> (w457:i8)
                          n188 = Increment(x=w457) -> (x+1=w456:i8)
                          n189 = local write "Counter"(w456) -> ()
                        }
                        frame True {
                        }
                      }
                      n190 = local write "Read?"(FALSE ("Read?")) -> ()
                      n191 = Number To Fractional String(number=w446, precision (6)=i16 3) -> (F-format string=w451:string)  [unwired: 2 in]
                      n192 = local read "Lake Shore"() -> (w449:refnum<visa-resource-name>)
                      n193 = Concatenate Strings("SETP 1," ("write buffer"), w451) -> (w453:string)
                      n194 = VISA Write(VISA resource name=w449, write buffer=w453, error in (no error)=w448) -> (error out=w447:errorcluster)  [unwired: 2 out]
                    }
                    frame False {
                      n195 = Equal?(x=w463, y=w460) -> (x = y?=w461:bool)
                      n196 = case shown="True" w461 {
                        tunnel: [w465 w468] -> w464
                        tunnel: w462 -> [_ w467]
                        tunnel: w459 -> [w465 w469]
                        frame False {
                        }
                        frame True {
                          # "Ramp Dn"
                          n197 = local write "Up/Down"(TRUE ("Up/Down")) -> ()
                          n198 = Number To Fractional String(number=w467, precision (6)=i16 3) -> (F-format string=w471:string)  [unwired: 2 in]
                          n199 = local read "Lake Shore"() -> (w466:refnum<visa-resource-name>)
                          n200 = Concatenate Strings("SETP 1," ("write buffer"), w471) -> (w473:string)
                          n201 = VISA Write(VISA resource name=w466, write buffer=w473, error in (no error)=w469) -> (error out=w468:errorcluster)  [unwired: 2 out]
                        }
                      }
                      n202 = local write "Read?"(FALSE ("Read?")) -> ()
                    }
                  }
                }
              }
              n203 = local read "Magnet"() -> (w365:bool)
              n204 = case shown="True" w365 {
                tunnel: [Mode."StepDelta" ("Enum") Mode."StepDelta" ("Enum")] -> w367
                frame False {
                }
                frame True {
                }
              }
            }
            frame "StepOxford" {
              n205 = local read "Actual Field (T)"() -> (w476:dbl)
              n206 = local read "Min Field (T)"() -> (w475:dbl)
              n207 = local read "Max Field (T)"() -> (w480:dbl)
              n208 = local read "Read?"() -> (w479:bool)
              n209 = Greater Or Equal?(x=w475, y=w476) -> (x >= y?=w478:bool)
              n210 = Compound Arithmetic op=AND(w478, w479) -> (w477:bool)
              n211 = case shown="True" w477 {
                tunnel: w480 -> [w488 w512]
                tunnel: w475 -> [_ w511]
                tunnel: w476 -> [_ w509]
                frame True {
                  # "Ramp Up"
                  n212 = local read "First?"() -> (w491:bool)
                  n213 = case shown="False" w491 {
                    tunnel: [TRUE ("Save") FALSE ("Save")] -> w489
                    tunnel: [w502 w506] -> w494
                    frame False {
                      n214 = local read "Counter"() -> (w505:i8)
                      n215 = local write "Actual Polarization"(0.0 ("Actual Polarization")) -> ()
                      n216 = Increment(x=w505) -> (x+1=w502:i8)
                      n217 = local write "Counter"(w502) -> ()
                    }
                    frame True {
                      (unwired) FALSE ("First?")
                      n218 = local read "Counter"() -> (w506:i8)
                      n219 = local read item#-1() -> ()  [unwired: 1 in]
                    }
                  }
                  n220 = local write "Read?"(FALSE ("Read?")) -> ()
                  n221 = local write "Up/Down"(FALSE ("Up/Down")) -> ()
                  n222 = local read "Record ALL"() -> (w492:bool)
                  n223 = case shown="True" w492 {
                    tunnel: w494 -> [_ w499]
                    tunnel: [FALSE w498] -> w493
                    frame False {
                    }
                    frame True {
                      n224 = local read "Max Countl"() -> (w497:i32)
                      n225 = Greater?(x=w499, y=w497) -> (0:w498:bool)
                    }
                  }
                  n226 = local write "Reset"(w489) -> ()
                  n227 = case shown="True" w493 {
                    tunnel: w488 -> [w500 _]
                    frame False {
                      n228 = local write "Target Field"(w500) -> ()
                    }
                    frame True {
                      n229 = local write "New"(TRUE) -> ()
                    }
                  }
                }
                frame False {
                  n230 = Less Or Equal?(x=w512, y=w509) -> (x <= y?=w510:bool)
                  n231 = case shown="True" w510 {
                    tunnel: w511 -> [_ w513]
                    frame False {
                    }
                    frame True {
                      # "Resetting at the end of every cycle"
                      # "Ramp Dn"
                      n232 = local write "Up/Down"(TRUE ("Up/Down")) -> ()
                      n233 = local write "Reset"(TRUE ("Reset")) -> ()
                      n234 = local write "Target Field"(w513) -> ()
                    }
                  }
                  n235 = local write "Read?"(FALSE ("Read?")) -> ()
                }
              }
            }
            frame "StepDelta" {
              n236 = flat-sequence {
                tunnel: w519 -> [w533]
                tunnel: [w532] -> w518
                frame #0 {
                  # "Check if it is time to step Field"
                  n237 = local read "Sweep Rate (T/min)"() -> (w534:dbl)
                  n238 = local read "B/V (T/V)"() -> (w526:dbl)
                  n239 = local read "Time Lag"() -> (w530:dbl)
                  n240 = xnode "Sweep Delay"("SweepRate"=w534, "Resolution"=0.001 ("Voltage Step (V)"), "BpV"=w526) -> ("Result"=w531:dbl)  [unwired: 1 in, 1 out]
                  n241 = Divide(x=w530, y=w531) -> (x/y=w528:dbl)
                  n242 = Multiply(x=0.001 ("y"), y=w528) -> (x*y=w527:dbl)
                  "deltaUaux" <- w527
                  n243 = stacked-sequence {
                    tunnel: w533 -> [_ w558]
                    tunnel: [_ w557] -> w532
                    tunnel: w527 -> [w536 _]
                    frame #0 {
                      n244 = local read "Actual Voltage (V)"() -> (w541:dbl)
                      n245 = local read "Up/Down"() -> (w542:bool)
                      n246 = Add(x=w541, y=w536) -> (x+y=w538:dbl)
                      n247 = Subtract(x=w541, y=w536) -> (x-y=w537:dbl)
                      n248 = Select(t=w537, s=w542, f=w538) -> (s? t:f=w540:dbl)
                      "Actual Voltage (V)" <- w540
                      n249 = local read "V/I (Ohm)"() -> (w543:dbl)
                      n250 = local read "B/V (T/V)"() -> (w544:dbl)
                      n251 = xnode "AUXtoB"("BpV"=w544, "Rm"=w543, "Aux"=w540) -> ("Result"=w539:dbl)  [unwired: 1 in, 1 out]
                      n252 = local write "Actual Field (T)"(w539) -> ()
                    }
                    frame #1 {
                      n253 = local read "Actual Voltage (V)"() -> (w563:dbl)
                      n254 = local read "Lock_in_Amplifier"() -> (w559:refnum<visa-resource-name>)
                      n255 = Format Into String(w563) -> (resulting string=w562:string)  [unwired: 3 in, 1 out]
                      n256 = Concatenate Strings("AUXV 1,", w562) -> (w560:string)
                      n257 = VISA Write(VISA resource name=w559, write buffer=w560, error in (no error)=w558) -> (error out=w557:errorcluster)  [unwired: 2 out]
                    }
                  }
                }
              }
            }
            frame "Plot" {
              # "dI"
              n258 = local read "P(uC/mm^2)"() -> (w577:dbl[])
              n259 = local read "Actual Polarization"() -> (w576:dbl)
              n260 = local read "Actual Current (pA)"() -> (w578:dbl)
              n261 = local read "Time Lag"() -> (w590:dbl)
              n262 = Multiply(x=w578, y=w590) -> (x*y=w582:dbl)
              n263 = Divide(x=w582, y="Sample area (mm^2)") -> (x/y=w581:dbl)
              n264 = Add(x=w581, y=w576) -> (x+y=w580:dbl)
              "Actual Polarization" <- w580
              n265 = local read "Temp/Magnetic Field"() -> (w591:bool)
              n266 = Build Array (concatenate)(w577, w580) -> (→"P(uC/mm^2)":dbl[])
              n267 = case shown="False" w591 {
                tunnel: w588 -> [_ w651]
                tunnel: w585 -> [_ w633]
                tunnel: w580 -> [w598 w634]
                frame False {
                  # "Magnetic Field plotting"
                  n268 = local read "Up/Down"() -> (w603:bool)
                  n269 = case shown="True" w603 {
                    frame True {
                      # "Down"
                      n270 = local read "I(B) 3"() -> (w613:cluster{dbl[], dbl[]}[])
                      n271 = local read "I(B) 3"() -> (w617:cluster{dbl[], dbl[]}[])
                      n272 = Index Array(array=w613, index=1) -> (element=w611:cluster{dbl[], dbl[]})
                      n273 = Unbundle(w611) -> (w610:dbl[], w609:dbl[])
                      n274 = Index Array(array=w617, index=i8 0 ("t")) -> (element=w614:cluster{dbl[], dbl[]})
                      n275 = local read "Actual Current (pA)"() -> (w604:dbl)
                      n276 = local read "Actual B Field (T)"() -> (w606:dbl)
                      n277 = Build Array (concatenate)(w610, w606) -> (w608:dbl[])
                      n278 = Build Array (concatenate)(w609, w604) -> (w607:dbl[])
                      n279 = Bundle(w608, w607) -> (w605:cluster{dbl[], dbl[]})  [unwired: 1 in]
                      n280 = Build Array(w614, w605) -> (w615:cluster{dbl[], dbl[]}[])
                      n281 = local write "I(B) 3"(w615) -> ()
                    }
                    frame False {
                      # "Up"
                      n282 = local read "I(B) 3"() -> (w629:cluster{dbl[], dbl[]}[])
                      n283 = local read "I(B) 3"() -> (w631:cluster{dbl[], dbl[]}[])
                      n284 = Index Array(array=w629, index=0) -> (element=w627:cluster{dbl[], dbl[]})
                      n285 = Unbundle(w627) -> (w626:dbl[], w625:dbl[])
                      n286 = Index Array(array=w631, index=i8 1 ("t")) -> (element=w620:cluster{dbl[], dbl[]})
                      n287 = local read "Actual B Field (T)"() -> (w621:dbl)
                      n288 = Build Array (concatenate)(w626, w621) -> (w624:dbl[])
                      n289 = local read "Actual Current (pA)"() -> (w618:dbl)
                      n290 = Build Array (concatenate)(w625, w618) -> (w623:dbl[])
                      n291 = Bundle(w624, w623) -> (w622:cluster{dbl[], dbl[]})  [unwired: 1 in]
                      n292 = Build Array(w622, w620) -> (w619:cluster{dbl[], dbl[]}[])
                      n293 = local write "I(B) 3"(w619) -> ()
                    }
                  }
                  n294 = local read "Actual B Field (T)"() -> (w600:dbl)
                  n295 = local read "P(B)"() -> (w602:cluster{"yi":dbl[], dbl[]})
                  n296 = Unbundle(w602) -> ("yi"=w601:dbl[], w599:dbl[])
                  n297 = Build Array (concatenate)(w601, w600) -> (w597:dbl[])
                  n298 = Build Array (concatenate)(w599, w598) -> (w596:dbl[])
                  n299 = Bundle(w597, w596) -> (→"P(B)":cluster{dbl[], dbl[]})  [unwired: 1 in]
                }
                frame True {
                  # "Temperature plotting"
                  n300 = Quotient & Remainder(x=w651, y="Save Period") -> (x-y*floor(x/y)=w632:dbl)  [unwired: 1 out]
                  n301 = Greater?(x=w633, y=w632) -> (0:w649:bool)
                  n302 = local read "Actual Temperature (K)"() -> (w636:dbl)
                  n303 = local read "Actual Current (pA)"() -> (w642:dbl)
                  n304 = local read "P(T)"() -> (w638:cluster{"yi":dbl[], dbl[]})
                  n305 = local read "I(T)"() -> (w648:cluster{dbl[], dbl[]})
                  n306 = case shown="True" w649 {
                    frame False {
                    }
                    frame True {
                      n307 = local write "Reset"(TRUE) -> ()
                    }
                  }
                  n308 = Unbundle(w638) -> ("yi"=w639:dbl[], w635:dbl[])
                  n309 = Unbundle(w648) -> (w646:dbl[], w645:dbl[])
                  n310 = Build Array (concatenate)(w639, w636) -> (w640:dbl[])
                  n311 = Build Array (concatenate)(w635, w634) -> (w641:dbl[])
                  n312 = Build Array (concatenate)(w646, w636) -> (w644:dbl[])
                  n313 = Build Array (concatenate)(w645, w642) -> (w643:dbl[])
                  n314 = Bundle(w644, w643) -> (→"I(T)":cluster{dbl[], dbl[]})  [unwired: 1 in]
                  n315 = Bundle(w640, w641) -> (→"P(T)":cluster{dbl[], dbl[]})  [unwired: 1 in]
                }
              }
            }
            frame "Save" {
              n316 = local read "Reset"() -> (w653:bool)
              n317 = case shown="False" w653 {
                tunnel: w658 -> [w675 w677]
                tunnel: [w675 w680] -> w663
                tunnel: w657 -> [w674 w678]
                tunnel: [w674 w680] -> w662
                tunnel: w659 -> [w673 w679]
                tunnel: [w673 w680] -> w661
                tunnel: [w672 w680] -> w660
                tunnel: w656 -> [w672 w676]
                frame False {
                }
                frame True {
                  n318 = stacked-sequence {
                    tunnel: [_ _ w732] -> w680
                    tunnel: w679 -> [_ w721 _]
                    tunnel: w678 -> [w707 w719 _]
                    tunnel: w677 -> [w708 w720 _]
                    tunnel: w676 -> [w697 w717 _]
                    frame #0 {
                      n319 = local read "B array"() -> (w691:dbl[])
                      n320 = local read "Counter"() -> (w706:i8)
                      n321 = local read "Averaged I(B)"() -> (w681:dbl[][])
                      n322 = local read "Up/Down"() -> (w709:bool)
                      n323 = local read "Sample area (mm^2)"() -> (w687:dbl)
                      n324 = call "Average_IBP_curves_baseline.vi"("I in"=w707, "Averaged P(B) In"="Averaged P(B)", "Counter"=w706, "B0"="Threshold B (T)", "Averaged I(B) In"=w681, "t in"=w697, "B in"=w708, "Averaged dt in"="Averaged dt", "Up/Down"=w709, "Sample area(mm^2)"=w687, "B array"=w691) -> ("Averaged I(B) out"=→"Averaged I(B)":dbl[][], "Averaged dt Out"=w694:dbl[][], "Averaged P(B) Out"=w683:dbl[][], "BaselineSubtracted I(B)"=w682:dbl[][])  [unwired: 1 in]
                      n325 = Index Array(array=w683, index (row)=0 ("disabled index (col)")) -> (element=w692:dbl[])  [unwired: 1 in]
                      n326 = Index Array(array=w683, index (row)=1 ("disabled index (col)")) -> (element=w693:dbl[])  [unwired: 1 in]
                      n327 = Index Array(array=w682, index (row)=0 ("disabled index (col)")) -> (element=w699:dbl[])  [unwired: 1 in]
                      n328 = Index Array(array=w682, index (row)=1 ("disabled index (col)")) -> (element=w698:dbl[])  [unwired: 1 in]
                      n329 = local write "Averaged dt"(w694) -> ()
                      n330 = Bundle("B array"=w691, "Averaged P(B) Out"=w692) -> (w690:T7)  [unwired: 1 in]
                      n331 = Bundle("B array"=w691, "Averaged P(B) Out"=w693) -> (w689:T7)  [unwired: 1 in]
                      n332 = local write "Averaged P(B)"(w683) -> ()
                      n333 = Bundle("B array"=w691, "BaselineSubtracted I(B)"=w699) -> (w705:T8)  [unwired: 1 in]
                      n334 = Bundle("B array"=w691, "BaselineSubtracted I(B)"=w698) -> (w704:T8)  [unwired: 1 in]
                      n335 = Build Array(w690, w689) -> (→"P(B) /Averaged/":T9)
                      n336 = Build Array(w705, w704) -> (→"I(B) /Averaged/":T10)
                    }
                    frame #1 {
                      # "Save and Reset"
                      n337 = local read "Temp/Magnetic Field"() -> (w710:bool)
                      n338 = local read "Measurement File"() -> (w712:path)
                      n339 = local read "P(uC/mm^2)"() -> (w718:dbl[])
                      n340 = Build Array(w721, w720, w719, w717, w718) -> (w711:dbl[][])
                      n341 = case shown="False" w710 {
                        tunnel: w712 -> [_ _]
                        tunnel: w711 -> [w726 _]
                        frame False {
                          n342 = local read "Up/Down"() -> (w724:bool)
                          n343 = case shown="False" w724 {
                            tunnel: [w729 w730] -> w723
                            frame False {
                              n344 = local read "Measurement File_dn"() -> (w729:path)
                            }
                            frame True {
                              n345 = local read "Measurement File_up"() -> (w730:path)
                            }
                          }
                          n346 = call-poly <vilib>:"Write Delimited Spreadsheet.vi"("file path (dialog if empty)"=w723, "format (%.3f)"="%.5g", "2D data"=w726, "append to file? (F)"=TRUE ("transpose? (F)"), "transpose? (F)"=FALSE ("append to file? (F)")) -> ()  [unwired: 9 in, 2 out]
                        }
                        frame True {
                        }
                      }
                      n347 = case shown="False" "Reset IB?" {
                        frame False {
                        }
                        frame True {
                          n348 = local read "Up/Down"() -> (w731:bool)
                          n349 = case shown="False" w731 {
                            frame False {
                              n350 = invoke on="I(B) 3" class="XYGraph (strict)" method="Reinit To Default"() -> ()  [unwired: 3 in, 3 out]
                            }
                            frame True {
                            }
                          }
                        }
                      }
                      n351 = call-poly <vilib>:"Write Delimited Spreadsheet.vi"("file path (dialog if empty)"=w712, "format (%.3f)"="%.5g", "2D data"=w711, "append to file? (F)"=TRUE, "transpose? (F)"=TRUE) -> ()  [unwired: 9 in, 2 out]
                      n352 = local write "Reset"(FALSE ("Save")) -> ()
                    }
                    frame #2 {
                      w732 = dbl[] []
                      n353 = local write "P(uC/mm^2)"(w732) -> ()
                    }
                  }
                }
              }
              n354 = local read "New"() -> (w655:bool)
              n355 = case shown="False" w655 {
                tunnel: [Mode."Return" ("Enum") Mode."New" ("Enum")] -> w667
                tunnel: [TRUE FALSE] -> w654
                frame False {
                }
                frame True {
                }
              }
            }
            frame "New" {
              n356 = stacked-sequence {
                seq-local: [_ _ _ _ w834 _ _] -> [_ _ _ _ _ w843 _]
                seq-local: [_ _ w788 _ _ _ _] -> [_ _ _ _ w833 _ _]
                tunnel: T6 {"Com Port"=1, "ISOBUS Address"=0, "GPIB Address"=25, "Communication"=enum."GPIB"} ("Address") -> [_ _ w787 w828 _ _ _]
                tunnel: w735 -> [_ _ w789 _ _ w844 _]
                tunnel: [_ _ _ _ _ w846 _] -> w734
                tunnel: w733 -> [_ w768 _ _ _ _ _]
                frame #0 {
                  w761 = 1 ("index (row)")
                  w760 = 0 ("index (row)")
                  # "Save averages"
                  n357 = local read "Measurement File_average"() -> (w748:path)
                  n358 = local read "Averaged P(B)"() -> (w759:dbl[][])
                  n359 = local read "Averaged dt"() -> (w757:dbl[][])
                  n360 = local read "I(B) /Averaged/"() -> (w749:cluster{"B array":dbl[], dbl[]}[])
                  n361 = Index Array(array=w757, index (row)=w760) -> (element=w758:dbl[])  [unwired: 1 in]
                  n362 = Index Array(array=w757, index (row)=w761) -> (element=w765:dbl[])  [unwired: 1 in]
                  n363 = Index Array(array=w749, index=1) -> (element=w753:cluster{"B array":dbl[], dbl[]})
                  n364 = Index Array(array=w749, index=0) -> (element=w752:cluster{"B array":dbl[], dbl[]})
                  n365 = Unbundle(w753) -> ("B array"=w763:dbl[], w764:dbl[])
                  n366 = Unbundle(w752) -> ("B array"=w754:dbl[], w755:dbl[])
                  n367 = Index Array(array=w759, index (row)=w760) -> (element=w762:dbl[])  [unwired: 1 in]
                  n368 = Index Array(array=w759, index (row)=w761) -> (element=w766:dbl[])  [unwired: 1 in]
                  n369 = Build Array(w754, w755, w758, w762, w763, w764, w765, w766) -> (w756:dbl[][])
                  n370 = call-poly <vilib>:"Write Delimited Spreadsheet.vi"("file path (dialog if empty)"=w748, "format (%.3f)"="%.5g", "2D data"=w756, "append to file? (F)"=TRUE ("transpose? (F)"), "transpose? (F)"=TRUE ("append to file? (F)")) -> ()  [unwired: 9 in, 2 out]
                }
                frame #1 {
                  w774 = dbl[] []
                  w783 = dbl[] []
                  # "Reset Flags"
                  n371 = Get Date/Time In Seconds() -> (seconds since 1Jan1904=w784:timestamp)
                  n372 = local write "Up/Down"(TRUE ("Up/Down")) -> ()
                  n373 = local write "First?"(TRUE ("First?")) -> ()
                  n374 = local write "Offset?"(FALSE ("Offset?")) -> ()
                  n375 = local write "New"(FALSE ("New")) -> ()
                  n376 = local write "P(uC/mm^2)"(w783) -> ()
                  n377 = local write "Start time"(w784) -> ()
                  n378 = local write "Offset array"(w783) -> ()
                  n379 = local write "Actual Polarization"(0.0 ("Actual Polarization")) -> ()
                  n380 = local write "Up/Down"(TRUE ("Up/Down")) -> ()
                  n381 = local write "Reset"(FALSE ("Reset")) -> ()
                  n382 = local read "B array"() -> (w777:dbl[])
                  n383 = local write "Counter"(i8 0 ("Counter")) -> ()
                  n384 = invoke on="P(B)" class="XYGraph (strict)" method="Reinit To Default"() -> ()  [unwired: 3 in, 3 out]
                  n385 = invoke on="I(B) 3" class="XYGraph (strict)" method="Reinit To Default"() -> ()  [unwired: 3 in, 3 out]
                  n386 = Multiply(x=w777, y=0.0) -> (x*y=w778:dbl[])
                  n387 = Build Array(w774, w774) -> (w782:dbl[][])
                  n388 = Bundle("B array"=w777, w778) -> (w779:cluster{"B array":dbl[], dbl[]})  [unwired: 1 in]
                  n389 = local write "Averaged I(B)"(w782) -> ()
                  n390 = Build Array(w779, w779) -> (w780:cluster{"B array":dbl[], dbl[]}[])
                  n391 = local write "I(B) /Averaged/"(w780) -> ()
                  n392 = local write "Measuring"(FALSE ("Measuring")) -> ()
                  n393 = Flush Queue(queue=w768) -> (remaining elements=→"remaining elements 2":T1)  [unwired: 1 in, 2 out]
                }
                frame #2 {
                  # "Step"
                  n394 = local read "Sweep Rate Array"() -> (w793:dbl[])
                  n395 = local read "j"() -> (w794:i32)
                  n396 = Increment(x=w794) -> (x+1=w790:i32)
                  n397 = Array Size(array=w793) -> (size(s)=w792:i32)
                  n398 = Less?(x=w790, y=w792) -> (x < y?=w791:bool)
                  "Step Rate" <- w791
                  n399 = case shown="True" w791 {
                    tunnel: w790 -> [_ w821]
                    tunnel: w789 -> [w797 w820]
                    tunnel: [w796 w820] -> w788
                    tunnel: w787 -> [w795 _]
                    frame False {
                      # "Step Temp?"
                      n400 = local read "Temperature Array"() -> (w801:dbl[])
                      n401 = local read "i"() -> (w802:i32)
                      n402 = Increment(x=w802) -> (x+1=w799:i32)
                      n403 = local write "j"(0 ("f")) -> ()
                      n404 = Array Size(array=w801) -> (size(s)=w800:i32)
                      n405 = Less?(x=w799, y=w800) -> (x < y?=w798:bool)
                      "Step Temp" <- w798
                      n406 = case shown="False" w798 {
                        tunnel: w799 -> [_ w819]
                        tunnel: w797 -> [w807 w818]
                        tunnel: [w806 w818] -> w796
                        tunnel: w795 -> [w805 _]
                        frame False {
                          # "Heater OFF"
                          # "Finished"
                          n407 = local write "i"(0 ("i")) -> ()
                          n408 = stacked-sequence {
                            tunnel: w807 -> [w811 _ _]
                            tunnel: [w810 _ _] -> w806
                            tunnel: w805 -> [_ w815 w816]
                            frame #0 {
                              n409 = local read "Lake Shore"() -> (w812:refnum<visa-resource-name>)
                              n410 = VISA Write(VISA resource name=w812, write buffer="RANGE,1,0", error in (no error)=w811) -> (error out=w810:errorcluster)  [unwired: 2 out]
                            }
                            frame #1 {
                              n411 = call "ips_switchHeaterOff.vi"("Instrument address"=w815, "Rate"=2.0) -> ()  [unwired: 1 out]
                            }
                            frame #2 {
                              n412 = call "GPIB - BusCommand.vi"("Command"="H0", "Address"=w816) -> ()  [unwired: 2 out]
                            }
                          }
                          n413 = local write "Record ALL"(FALSE ("Record ALL")) -> ()
                          "Finished" <- TRUE
                        }
                        frame True {
                          n414 = local write "i"(w819) -> ()
                        }
                      }
                    }
                    frame True {
                      n415 = local write "j"(w821) -> ()
                    }
                  }
                }
                frame #3 {
                  # "Set rates"
                  n416 = local read "Sweep Rate Array"() -> (w827:dbl[])
                  n417 = local read "j"() -> (w826:i32)
                  n418 = local read "j"() -> (w824:i32)
                  n419 = Index Array(array=w827, index=w826) -> (element=w825:dbl)
                  n420 = Number To Fractional String(number=w825, precision (6)=i16 3) -> (F-format string=w831:string)  [unwired: 2 in]
                  n421 = Index Array(array="Max count array", index=w824) -> (element=w822:i32)
                  n422 = local write "Max Countl"(w822) -> ()
                  n423 = Concatenate Strings("T" ("format string"), w831) -> (w832:string)
                  n424 = call "GPIB - BusCommand.vi"("Command"=w832, "Address"=w828) -> ()  [unwired: 2 out]
                  n425 = local write "Sweep Rate (T/min)"(w825) -> ()
                }
                frame #4 {
                  # "Set temperature"
                  n426 = local read "Temperature Array"() -> (w837:dbl[])
                  n427 = local read "i"() -> (w836:i32)
                  n428 = Index Array(array=w837, index=w836) -> (element=w835:dbl)
                  n429 = local read "Lake Shore"() -> (w839:refnum<visa-resource-name>)
                  n430 = Number To Fractional String(number=w835, precision (6)=i16 3) -> (F-format string=w840:string)  [unwired: 2 in]
                  n431 = Concatenate Strings("SETP 1," ("write buffer"), w840) -> (w842:string)
                  n432 = VISA Write(VISA resource name=w839, write buffer=w842, error in (no error)=w833) -> (error out=w834:errorcluster)  [unwired: 2 out]
                }
                frame #5 {
                  n433 = local read "Finished"() -> (w845:bool)
                  n434 = case shown="False" w845 {
                    tunnel: [w859 w896] -> w846
                    tunnel: w844 -> [_ _]
                    tunnel: w843 -> [w856 w896]
                    frame False {
                      w854 = "_" ("string")
                      # "Wait, create Files"
                      n435 = local read "Temperature Array"() -> (w886:dbl[])
                      n436 = local read "Sweep Rate Array"() -> (w882:dbl[])
                      n437 = local read "i"() -> (w885:i32)
                      n438 = local read "j"() -> (w883:i32)
                      n439 = Index Array(array=w886, index=w885) -> (element=w884:dbl)
                      n440 = Index Array(array=w882, index=w883) -> (element=w851:dbl)
                      n441 = Round Toward -Infinity(1:w851) -> (0:w852:dbl)
                      n442 = Number To Fractional String(use system decimal point (T)=TRUE, number=w884, precision (6)=i16 1) -> (F-format string=w887:string)  [unwired: 1 in]
                      n443 = Subtract(x=w851, y=w852) -> (x-y=w853:dbl)
                      n444 = Equal To 0?(x=w853) -> (x = 0?=w850:bool)
                      n445 = Select(t=i16 0 ("precision (6)"), s=w850, f=i16 2 ("precision (6)")) -> (s? t:f=w847:i16)
                      n446 = Number To Fractional String(use system decimal point (T)=TRUE, number=w851, precision (6)=w847) -> (F-format string=w855:string)  [unwired: 1 in]
                      n447 = Concatenate Strings("Directory", "\\" ("string"), "FileName", w854, w887, "K" ("string"), w854, w855, "Tpm" ("string")) -> (w876:string)
                      n448 = Search and Replace String(replace all?=TRUE ("replace all? (F)"), input string=w876, search string=".", replace string="p" ("substring (\"\")"), error in=w856) -> (result string=w871:string, error out=w866:errorcluster)  [unwired: 3 in, 2 out]
                      n449 = local write "Step Rate"(FALSE ("Step Rate")) -> ()
                      n450 = Concatenate Strings(w871, ".txt" ("string")) -> (w870:string)
                      n451 = local read "Step Temp"() -> (w860:bool)
                      n452 = String To Path(string=w870) -> (path=w869:path)
                      n453 = Open/Create/Replace File(file path (use dialog)=w869, error in=w866, operation (0:open)=T5."open or create") -> (refnum out=w858:refnum<file>, error out=w859:errorcluster)  [unwired: 3 in, 1 out]
                      n454 = local write "refnum out"(w858) -> ()
                      n455 = Refnum to Path(1:w858) -> (0:w861:path)
                      n456 = call "Create_sweep_files.vi"("Measurement File"=w861) -> ("Path 3"=w864:path, "Path 2"=w863:path, "Path"=w862:path)  [unwired: 8 in]
                      n457 = local write "Measurement File"(w861) -> ()
                      n458 = case shown="True" w860 {
                        frame False {
                        }
                        frame True {
                          n459 = Get Date/Time In Seconds() -> (seconds since 1Jan1904=w889:timestamp)
                          n460 = local write "Step Temp"(FALSE ("Step Temp")) -> ()
                          n461 = while {
                            tunnel: w889 -> [w894]
                            stop <- w891 stop-if-true
                            n462 = Get Date/Time In Seconds() -> (seconds since 1Jan1904=w895:timestamp)
                            n463 = Subtract(x=w895, y=w894) -> (x-y=w893:dbl)
                            "Wait (s)" <- w893
                            n464 = Greater Or Equal?(x=w893, y="secs to wait") -> (x >= y?=w891:bool)
                          }
                        }
                      }
                      n465 = local write "Measurement File_dn"(w864) -> ()
                      n466 = local write "Measurement File_average"(w862) -> ()
                      n467 = local write "Measurement File_up"(w863) -> ()
                    }
                    frame True {
                    }
                  }
                }
                frame #6 {
                  n468 = local read "Finished"() -> (w897:bool)
                  n469 = case shown="True" w897 {
                    frame False {
                      n470 = local write "Measuring"(TRUE ("Measuring")) -> ()
                    }
                    frame True {
                      n471 = local write "Measure /Pause"(FALSE ("Measure /Pause")) -> ()
                    }
                  }
                }
              }
            }
            frame "Return" {
            }
          }
        }
      }
      frame Error {
        # "Return true for any case which should stop the loop."
      }
    }
  }
  n472 = case shown="True" w51 {
    frame False {
    }
    frame True {
      n473 = local read "B array"() -> (w920:dbl[])
      n474 = invoke on="P(T)" class="XYGraph (strict)" method="Reinit To Default"() -> ()  [unwired: 3 in, 3 out]
      n475 = invoke on="I(T)" class="XYGraph (strict)" method="Reinit To Default"() -> ()  [unwired: 3 in, 3 out]
      n476 = invoke on="P(B)" class="XYGraph (strict)" method="Reinit To Default"() -> ()  [unwired: 3 in, 3 out]
      n477 = invoke on="I(B) 3" class="XYGraph (strict)" method="Reinit To Default"() -> ()  [unwired: 3 in, 3 out]
      n478 = Multiply(x=w920, y=0.0) -> (x*y=w919:dbl[])
      n479 = Bundle("B array"=w920, w919) -> (w918:cluster{"B array":dbl[], dbl[]})  [unwired: 1 in]
      n480 = Build Array(w918, w918) -> (w917:cluster{"B array":dbl[], dbl[]}[])
      n481 = local write "I(B) /Averaged/"(w917) -> ()
      n482 = invoke on="P(B) /Averaged/" class="XYGraph (strict)" method="Reinit To Default"() -> ()  [unwired: 3 in, 3 out]
    }
  }
  n483 = while {
    shift-right: [w934] -> w90
    shift-left: w71 -> [w935]
    shift-right: [w936] -> w97
    shift-left: w98 -> [w937]
    tunnel: w93 -> [w933]
    tunnel: w92 -> [w932]
    tunnel: w37 -> [w931]
    tunnel: [w925] -> _
    tunnel: w79 -> [w924]
    tunnel: w69 -> [w923]
    tunnel: w4 -> [w922]
    stop <- "stop" stop-if-true
    n484 = event shown="[0] Timeout" {
      selector: _ -> [_ _ _ _ _ _ _ _ _ _ _ _ _ _ _]
      dyn-events: _ -> [_ _ _ _ _ _ _ _ _ _ _ _ _ _ _]
      timeout: 10 -> [_ _ _ _ _ _ _ _ _ _ _ _ _ _ _]
      tunnel: w937 -> [w948 w994 w1004 w1018 w1089 w1093 w1097 w1137 w1153 w1170 w1213 w1230 w1246 w1256 w1267]
      tunnel: [w947 w994 w1004 w1018 w1089 w1093 w1097 w1137 w1153 w1170 w1213 w1230 w1246 w1256 w1267] -> w936
      tunnel: w935 -> [w946 w993 w1003 w1016 w1088 w1095 w1099 w1138 w1152 w1169 w1214 w1232 w1250 w1260 w1269]
      tunnel: [w945 w993 w1003 w1015 w1090 w1095 w1098 _ w1152 w1169 w1214 w1231 w1249 w1259 w1268] -> w934
      tunnel: w933 -> [w944 _ _ _ _ _ _ _ _ _ _ _ _ _ _]
      tunnel: w932 -> [w943 _ _ _ _ _ _ _ _ _ _ _ _ _ _]
      tunnel: w931 -> [w942 _ _ _ _ _ _ _ _ _ _ _ _ _ _]
      tunnel: [w940 w992 w1002 w1017 w1091 w1094 w1096 w1136 w1151 w1168 w1212 w1229 w1247 w1257 _] -> w925
      tunnel: w924 -> [w940 w992 w1005 w1017 w1091 w1094 w1096 w1136 w1151 w1168 w1212 w1229 w1247 w1257 _]
      tunnel: w923 -> [_ _ _ _ _ _ _ _ _ _ _ w1233 w1248 w1261 w1266]
      tunnel: [_ _ _ _ _ _ _ w1138 _ _ _ _ _ _ _] -> _
      tunnel: w922 -> [w939 _ _ _ _ _ _ _ _ _ _ _ _ _ _]
      event Timeout {
        n485 = event-data() -> ()  [unwired: 1 in, 3 out]
        n486 = case shown="True" "Measuring" {
          tunnel: w948 -> [w950 w973]
          tunnel: [w950 w972] -> w947
          tunnel: w946 -> [w949 _]
          tunnel: [w949 w971] -> w945
          tunnel: w944 -> [_ w964]
          tunnel: w943 -> [_ w963]
          tunnel: w942 -> [_ w959]
          tunnel: w939 -> [_ w953]
          frame False {
          }
          frame True {
            w962 = ":FETCh? " ("data")
            w965 = u32 1000 ("byte count")
            # "Generate the data here."
            n487 = case shown="No Error" w959 {
              selector: w959 -> [w985 w986]
              tunnel: [w985 w986] -> w958
              tunnel: [w984 _] -> w957
              frame No Error {
                n488 = Get Date/Time In Seconds() -> (seconds since 1Jan1904=w984:timestamp)
              }
              frame Error {
              }
            }
            n489 = VISA Write(VISA resource name=w964, write buffer=w962, error in (no error)=w958) -> (VISA resource name out=w970:refnum<visa-resource-name>, error out=w968:errorcluster)  [unwired: 1 out]
            n490 = VISA Write(VISA resource name=w963, write buffer=w962, error in (no error)=w968) -> (VISA resource name out=w969:refnum<visa-resource-name>, error out=w967:errorcluster)  [unwired: 1 out]
            n491 = VISA Read(VISA resource name=w970, byte count=w965, error in (no error)=w967) -> (read buffer=w960:string, error out=w966:errorcluster)  [unwired: 2 out]
            n492 = VISA Read(VISA resource name=w969, byte count=w965, error in (no error)=w966) -> (read buffer=w961:string, error out=w955:errorcluster)  [unwired: 2 out]
            n493 = case shown="False" "DaQ" {
              tunnel: w955 -> [w975 w981]
              tunnel: [w975 w980] -> w954
              tunnel: w953 -> [_ w979]
              tunnel: [0.0 ("Output") w977] -> w951
              frame False {
              }
              frame True {
                n494 = local read "Number of Samples"() -> (w983:i32)
                n495 = call-poly <vilib>:"DAQmx Read.vi"("task/channels in"=w979, "number of samples per channel"=w983, "error in"=w981) -> ("data"=w982:dbl[], "error out"=w980:errorcluster)  [unwired: 10 in, 1 out]
                n496 = call-poly <vilib>:"Mean.vi"("X"=w982) -> ("mean"=w978:dbl)  [unwired: 1 out]
                "Actual mean" <- w978
                n497 = call "N Point Running Average.vi"("n"="Moving average", "Input"=w978) -> ("Output"=w977:dbl)
              }
            }
            n498 = Bundle("seconds since 1Jan1904"=w957, "read buffer"=w960, "read buffer"=w961, "Output"=w951) -> (w956:T4)  [unwired: 1 in]
            n499 = Enqueue Element(queue=w973, element=w956, error in (no error)=w954) -> (queue out=w972:refnum<queue>, error out=w971:errorcluster)  [unwired: 1 in, 1 out]
          }
        }
      }
      event "Max Field (T)": Value Change {
        n500 = event-data() -> ()  [unwired: 1 in, 6 out]
        n501 = Divide(x="Max Field (T)", y="dB (T)") -> (x/y=w989:dbl)
        n502 = for {
          N: w989 -> [_]
          tunnel: "dB (T)" -> [w999]
          tunnel: [w996] -> w988 mode=indexing
          tunnel: "Min Field (T)" -> [w997]
          tunnel: [0.0] -> _ mode=indexing
          i -> [w1000]
          n503 = Multiply(x=w1000, y=w999) -> (x*y=w998:dbl)
          n504 = Add(x=w998, y=w997) -> (x+y=w996:dbl)
        }
        "B array" <- w988
      }
      event "Sweep Rate (T/min)": Value Change {
        n505 = event-data() -> ("NewVal"=w1006:dbl)  [unwired: 1 in, 5 out]
        n506 = local read "Magnet"() -> (w1001:bool)
        n507 = case shown="False" w1001 {
          tunnel: w1006 -> [_ w1013]
          tunnel: w1005 -> [w1007 w1009]
          tunnel: [w1007 w1008] -> w1002
          frame False {
          }
          frame True {
            n508 = Number To Fractional String(number=w1013, precision (6)=i16 3) -> (F-format string=w1011:string)  [unwired: 2 in]
            n509 = Concatenate Strings("T" ("format string"), w1011) -> (w1010:string)
            n510 = call "GPIB - BusCommand.vi"("Command"=w1010, "Address"=w1009) -> ("Address(thru)"=w1008:T6)  [unwired: 1 out]
          }
        }
      }
      event "Field To Zero": Value Change {
        n511 = event-data() -> ()  [unwired: 1 in, 6 out]
        n512 = Two Button Dialog(message="Do you want to switch off the field?", 1:"No" ("F button name (\"Cancel\")"), 2:"Yes" ("T button name (\"OK\")")) -> (T button?=w1022:bool)
        n513 = case shown="True" w1022 {
          tunnel: w1017 -> [_ w1027]
          tunnel: w1016 -> [w1023 w1025]
          tunnel: [w1023 w1024] -> w1015
          frame False {
          }
          frame True {
            n514 = local read "Magnet"() -> (w1026:bool)
            n515 = case shown="False" w1026 {
              tunnel: w1027 -> [_ w1079]
              tunnel: w1025 -> [w1030 w1076]
              tunnel: [w1029 w1076] -> w1024
              frame False {
                n516 = local read "Lock_in_Amplifier"() -> (w1028:refnum<visa-resource-name>)
                n517 = stacked-sequence {
                  seq-local: [w1033 _] -> [_ w1045]
                  seq-local: [w1031 _] -> [_ w1042]
                  tunnel: w1030 -> [w1035 _]
                  tunnel: [_ w1048] -> w1029
                  tunnel: w1028 -> [w1032 w1043]
                  frame #0 {
                    n518 = VISA Write(VISA resource name=w1032, write buffer="AUXV?1", error in (no error)=w1035) -> (VISA resource name out=w1039:refnum<visa-resource-name>, error out=w1034:errorcluster)  [unwired: 1 out]
                    n519 = VISA Read(VISA resource name=w1039, byte count=u32 1000, error in (no error)=w1034) -> (read buffer=w1036:string, error out=w1033:errorcluster)  [unwired: 2 out]
                    n520 = Fract/Exp String To Number(string=w1036) -> (number=w1031:dbl)  [unwired: 3 in, 1 out]
                  }
                  frame #1 {
                    w1051 = 0.001 ("Voltage Step (V)")
                    n521 = local read "Sweep Rate (T/min)"() -> (w1050:dbl)
                    n522 = local read "V/I (Ohm)"() -> (w1047:dbl)
                    n523 = local read "B/V (T/V)"() -> (w1041:dbl)
                    n524 = xnode "Sweep Delay"("SweepRate"=w1050, "Resolution"=w1051, "BpV"=w1041) -> ("Result"=w1049:dbl)  [unwired: 1 in, 1 out]
                    n525 = call "Universal_Ramping.vi"("milliseconds to wait"=w1049, "Initial Voltage (V)"=w1042, "error in (no error)"=w1045, "Voltage Step (V)"=w1051, "Final Voltage (V)"=0.0, "VISA resource name"=w1043) -> ("error out"=w1048:errorcluster, "Actual Voltage (V)"=w1040:dbl)  [unwired: 3 in, 1 out]
                    n526 = local write "Actual Voltage (V)"(w1040) -> ()
                    n527 = xnode "AUXtoB"("BpV"=w1041, "Rm"=w1047, "Aux"=w1040) -> ("Result"=w1046:dbl)  [unwired: 1 in, 1 out]
                    n528 = local write "Actual B Field (T)"(w1046) -> ()
                  }
                }
              }
              frame True {
                n529 = local read "Sweep Rate (T/min)"() -> (w1078:dbl)
                n530 = call "ips_switchHeaterOff.vi"("Instrument address"=w1079, "Rate"=w1078) -> ("B"=w1077:dbl)
                n531 = local write "Actual Field (T)"(w1077) -> ()
              }
            }
          }
        }
      }
      event "Go to Set": Value Change {
        n532 = event-data() -> ()  [unwired: 1 in, 6 out]
        n533 = local read "V/I (Ohm)"() -> (w1086:dbl)
        n534 = local read "B/V (T/V)"() -> (w1085:dbl)
        n535 = local read "Lock_in_Amplifier"() -> (w1082:refnum<visa-resource-name>)
        n536 = local read "Sweep Rate (T/min)"() -> (w1084:dbl)
        n537 = local read "Magnet"() -> (w1087:bool)
        n538 = call "Ramp_Field.vi"("Set Field (T) in"="Set Field (T)", "Sweep Rate (T/min)"=w1084, "V/I (Ohm)"=w1086, "error in (no error)"=w1088, "Magnet"=w1087, "B/V (T/V)"=w1085, "VISA Refnum in"=w1082) -> ("error out"=w1090:errorcluster, "Actual Voltage (V)"=w1080:dbl, "Set Field (T) out"=w1083:dbl)  [unwired: 2 in]
        n539 = local write "Actual B Field (T)"(w1083) -> ()
        n540 = local write "Actual Voltage (V)"(w1080) -> ()
      }
      event "Measure /Pause": Value Change {
        n541 = event-data() -> ("NewVal"=w1092:bool)  [unwired: 1 in, 5 out]
        n542 = local write "Measuring"(w1092) -> ()
      }
      event "Stop": Value Change {
        n543 = event-data() -> ()  [unwired: 1 in, 6 out]
        n544 = local read "Measuring"() -> (w1100:bool)
        n545 = case shown="True" w1100 {
          tunnel: w1099 -> [w1101 w1104]
          tunnel: [w1101 w1105] -> w1098
          frame False {
          }
          frame True {
            w1112 = FALSE ("Measuring")
            n546 = local read "SaveSweep"() -> (w1113:bool)
            n547 = local write "Measuring"(w1112) -> ()
            n548 = local write "Measure /Pause"(w1112) -> ()
            n549 = local read "Lock_in_Amplifier"() -> (w1106:refnum<visa-resource-name>)
            n550 = case shown="True" w1113 {
              frame False {
              }
              frame True {
                w1119 = 1 ("index (row)")
                w1120 = 0 ("index (row)")
                n551 = local read "Measurement File_average"() -> (w1132:path)
                n552 = local read "Averaged P(B)"() -> (w1121:dbl[][])
                n553 = local read "Averaged dt"() -> (w1123:dbl[][])
                n554 = local read "I(B) /Averaged/"() -> (w1131:cluster{"B array":dbl[], dbl[]}[])
                n555 = Index Array(array=w1123, index (row)=w1120) -> (element=w1122:dbl[])  [unwired: 1 in]
                n556 = Index Array(array=w1123, index (row)=w1119) -> (element=w1115:dbl[])  [unwired: 1 in]
                n557 = Index Array(array=w1131, index=1) -> (element=w1127:cluster{"B array":dbl[], dbl[]})
                n558 = Index Array(array=w1131, index=0) -> (element=w1128:cluster{"B array":dbl[], dbl[]})
                n559 = Unbundle(w1127) -> ("B array"=w1117:dbl[], w1116:dbl[])
                n560 = Unbundle(w1128) -> ("B array"=w1126:dbl[], w1125:dbl[])
                n561 = Index Array(array=w1121, index (row)=w1120) -> (element=w1118:dbl[])  [unwired: 1 in]
                n562 = Index Array(array=w1121, index (row)=w1119) -> (element=w1114:dbl[])  [unwired: 1 in]
                n563 = Build Array(w1126, w1125, w1122, w1118, w1117, w1116, w1115, w1114) -> (w1124:dbl[][])
                n564 = call-poly <vilib>:"Write Delimited Spreadsheet.vi"("file path (dialog if empty)"=w1132, "format (%.3f)"="%.5g", "2D data"=w1124, "append to file? (F)"=TRUE ("transpose? (F)"), "transpose? (F)"=TRUE ("append to file? (F)")) -> ()  [unwired: 9 in, 2 out]
              }
            }
            n565 = local read "V/I (Ohm)"() -> (w1110:dbl)
            n566 = local read "Sweep Rate (T/min)"() -> (w1109:dbl)
            n567 = local read "Set Field (T)"() -> (w1111:dbl)
            n568 = local read "B/V (T/V)"() -> (w1107:dbl)
            n569 = local read "Magnet"() -> (w1108:bool)
            n570 = call "Ramp_Field.vi"("Set Field (T) in"=w1111, "Sweep Rate (T/min)"=w1109, "V/I (Ohm)"=w1110, "error in (no error)"=w1104, "Magnet"=w1108, "B/V (T/V)"=w1107, "VISA Refnum in"=w1106) -> ("error out"=w1105:errorcluster, "Actual Voltage (V)"=w1102:dbl, "Set Field (T) out"=w1103:dbl)  [unwired: 2 in]
            n571 = local write "Actual B Field (T)"(w1103) -> ()
            n572 = local write "Actual Voltage (V)"(w1102) -> ()
          }
        }
      }
      event "Sweep": Value Change {
        n573 = event-data() -> ("NewVal"=w1139:bool)  [unwired: 1 in, 5 out]
        n574 = case shown="True" w1139 {
          frame False {
          }
          frame True {
            n575 = local read "Measurement File"() -> (w1140:path)
            n576 = Two Button Dialog(message="Do you want to create additional files for the sweeping measurements?" ("string"), 1:"No" ("F button name (\"Cancel\")"), 2:"Yes" ("T button name (\"OK\")")) -> (T button?=w1142:bool)
            n577 = case shown="True" w1142 {
              tunnel: w1140 -> [_ w1147]
              frame False {
                n578 = local write "SaveSweep"(FALSE ("SaveSweep")) -> ()
              }
              frame True {
                n579 = call "Create_sweep_files.vi"("Measurement File"=w1147) -> ("Path 3"=→"Measurement File_dn":path, "Path 2"=→"Measurement File_up":path, "Path"=→"Measurement File_average":path)  [unwired: 8 in]
                "SaveSweep" <- TRUE
              }
            }
          }
        }
      }
      event "Measure Noise": Value Change {
        n580 = event-data() -> ("NewVal"=w1154:bool)  [unwired: 1 in, 5 out]
        n581 = case shown="True" w1154 {
          frame False {
          }
          frame True {
            n582 = local read "Gain (V/A)"() -> (w1159:dbl)
            n583 = call "Noise_measurement.vi"("Gain (V/A)"=w1159, "Cycles"="Cycles", "Lower Cut-Off"="Cut-Off Frequency", "minimum value"="minimum value", "Filter On"="Filter On", "maximum value"="maximum value", "physical channels"="physical channels", "rate"="Rate", "samples per channel"="Samples per channel") -> ("Current (pA) Filtered"=→"Current (pA) Filtered":waveform(dbl), "PSD (pA/Hz^1/2) Peaks Removed"=→"PSD (pA/Hz^1/2) Peaks Removed":cluster{"f0":dbl, "df":dbl, "magnitude":dbl[]}, "Current (pA)"=→"Current (pA)":dbl[], "PSD (pA/Hz^1/2)"=→"PSD (pA/Hz^1/2)":cluster{"f0":dbl, "df":dbl, "magnitude":dbl[]})  [unwired: 3 in]
          }
        }
      }
      event "Calibrate": Value Change {
        n584 = event-data() -> ()  [unwired: 1 in, 6 out]
        n585 = case shown="True" "Calibrate" {
          frame False {
          }
          frame True {
            w1174 = dbl[] []
            n586 = while {
              shift-right: [w1207] -> w1172
              shift-left: dbl[][] [] -> [w1206]
              shift-right: [w1190] -> _
              shift-left: w1174 -> [w1202]
              shift-right: [w1199] -> _
              shift-left: w1174 -> [w1201]
              shift-right: [w1189] -> _
              shift-left: w1174 -> [w1200]
              shift-right: [w1181] -> _
              shift-left: 0.0 ("Set Field out") -> [w1180]
              stop <- w1203 stop-if-true
              n587 = call "Calibtarion.vi"("Dwell Time (ms)"="Dwell Time (ms)", "V array in (V)"=w1202, "I array in (A)"=w1200, "Collected array in"=w1206, "B array in (T)"=w1201, "Set Field (T)"=w1180, "dB"="dB") -> ("Best Linear Fit"=w1191:dbl[], "appended array"=→"appended array":dbl[][], "slope"=→"B/V (T/V)":dbl, "V array out (V)"=w1190:dbl[], "Boolean"=w1205:bool, "I array out (A)"=w1189:dbl[], "intercept 2"=→"I0 (A)":dbl, "Collected array out"=w1207:dbl[][], "intercept"=→"B0 (T)":dbl, "B array Out"=w1199:dbl[], "slope 2"=→"V/I (Ohm)":dbl, "Best Linear Fit 2"=w1196:dbl[], "Set Field out"=w1181:dbl)
              n588 = Bundle("I array out (A)"=w1189, "V array out (V)"=w1190) -> (w1198:T11)  [unwired: 1 in]
              n589 = Bundle("I array out (A)"=w1189, "Best Linear Fit"=w1191) -> (w1192:T12)  [unwired: 1 in]
              n590 = Bundle("V array out (V)"=w1190, "B array Out"=w1199) -> (w1194:T13)  [unwired: 1 in]
              n591 = Bundle("V array out (V)"=w1190, "Best Linear Fit 2"=w1196) -> (w1195:T14)  [unwired: 1 in]
              n592 = Or(x=w1205, y="stop 2") -> (x .or. y?=w1203:bool)
              n593 = Build Array(w1198, w1192) -> (→"V_I":T15)
              n594 = Build Array(w1194, w1195) -> (→"B_V":T16)
            }
            n595 = flat-sequence {
              tunnel: w1172 -> [w1178]
              frame #0 {
                n596 = Two Button Dialog(message="Do you want to save calibration file?") -> (T button?=w1177:bool)  [unwired: 2 in]
                n597 = case shown="True" w1177 {
                  tunnel: w1178 -> [_ w1179]
                  frame False {
                  }
                  frame True {
                    n598 = call-poly <vilib>:"Write Delimited Spreadsheet.vi"("2D data"=w1179) -> ()  [unwired: 13 in, 2 out]
                  }
                }
              }
            }
          }
        }
      }
      event "New Measurement File": Value Change {
        n599 = event-data() -> ()  [unwired: 1 in, 6 out]
        n600 = local read "Sweep"() -> (w1209:bool)
        n601 = Open/Create/Replace File(prompt="Please select measurement file\n", operation (0:open)=T5."replace or create with confirmation") -> (refnum out=w1215:refnum<file>)  [unwired: 4 in, 2 out]
        n602 = local write "refnum out"(w1215) -> ()
        n603 = Refnum to Path(1:w1215) -> (0:w1210:path)
        n604 = case shown="True" w1209 {
          tunnel: w1210 -> [_ w1218]
          frame False {
          }
          frame True {
            n605 = Two Button Dialog(message="Do you want to create additional files for the sweeping measurements?" ("string"), 1:"No" ("F button name (\"Cancel\")"), 2:"Yes" ("T button name (\"OK\")")) -> (T button?=w1220:bool)
            n606 = case shown="False" w1220 {
              tunnel: w1218 -> [_ w1228]
              frame False {
                n607 = local write "SaveSweep"(FALSE ("SaveSweep")) -> ()
              }
              frame True {
                n608 = call "Create_sweep_files.vi"("Measurement File"=w1228) -> ("Path 3"=w1225:path, "Path 2"=w1226:path, "Path"=w1227:path)  [unwired: 8 in]
                n609 = local write "Measurement File_dn"(w1225) -> ()
                n610 = local write "Measurement File_average"(w1227) -> ()
                n611 = local write "Measurement File_up"(w1226) -> ()
                n612 = local write "SaveSweep"(TRUE) -> ()
              }
            }
          }
        }
        n613 = local write "Measurement File"(w1210) -> ()
        n614 = local write "Offset?"(FALSE ("Offset?")) -> ()
        n615 = local write "First?"(TRUE ("First?")) -> ()
      }
      event "Heater On/Off": Value Change {
        n616 = event-data() -> ()  [unwired: 1 in, 6 out]
        n617 = case shown="False" "Heater On/Off" {
          tunnel: w1233 -> [w1238 w1244]
          tunnel: w1232 -> [w1236 w1245]
          tunnel: [w1235 w1243] -> w1231
          frame False {
            n618 = VISA Write(VISA resource name=w1238, write buffer="RANGE,1,0", error in (no error)=w1236) -> (error out=w1235:errorcluster)  [unwired: 2 out]
          }
          frame True {
            n619 = Number To Decimal String(number="Heater Range") -> (decimal integer string=w1241:string)  [unwired: 1 in]
            n620 = Concatenate Strings("RANGE,1," ("write buffer"), w1241) -> (w1239:string)
            n621 = VISA Write(VISA resource name=w1244, write buffer=w1239, error in (no error)=w1245) -> (error out=w1243:errorcluster)  [unwired: 2 out]
          }
        }
      }
      event "Set temperature (K)": Value Change {
        n622 = event-data() -> ()  [unwired: 1 in, 6 out]
        n623 = local read "Set temperature (K)"() -> (w1251:dbl)
        n624 = Number To Fractional String(number=w1251, precision (6)=i16 3) -> (F-format string=w1254:string)  [unwired: 2 in]
        n625 = Concatenate Strings("SETP 1," ("write buffer"), w1254) -> (w1252:string)
        n626 = VISA Write(VISA resource name=w1248, write buffer=w1252, error in (no error)=w1250) -> (error out=w1249:errorcluster)  [unwired: 2 out]
      }
      event "Temp Ramping Rate (K/min)": Value Change {
        n627 = event-data() -> ()  [unwired: 1 in, 6 out]
        n628 = local read "Temp Ramping Rate (K/min)"() -> (w1258:dbl)
        n629 = Number To Fractional String(number=w1258, precision (6)=i16 1) -> (F-format string=w1264:string)  [unwired: 2 in]
        n630 = Concatenate Strings("RAMP 1,1," ("string"), w1264) -> (w1263:string)
        n631 = VISA Write(VISA resource name=w1261, write buffer=w1263, error in (no error)=w1260) -> (error out=w1259:errorcluster)  [unwired: 2 out]
      }
      event "Heater Range": Value Change {
        n632 = event-data() -> ()  [unwired: 1 in, 6 out]
        n633 = local read "Heater On/Off"() -> (w1270:bool)
        n634 = case shown="True" w1270 {
          tunnel: w1269 -> [w1271 w1276]
          tunnel: [w1271 w1275] -> w1268
          tunnel: w1266 -> [_ w1274]
          frame False {
          }
          frame True {
            n635 = local read "Heater Range"() -> (w1272:enum16{"Off", "Low", "Medium", "High"})
            n636 = Number To Decimal String(number=w1272) -> (decimal integer string=w1278:string)  [unwired: 1 in]
            n637 = Concatenate Strings("RANGE,1," ("write buffer"), w1278) -> (w1277:string)
            n638 = VISA Write(VISA resource name=w1274, write buffer=w1277, error in (no error)=w1276) -> (error out=w1275:errorcluster)  [unwired: 2 out]
          }
        }
      }
    }
    n639 = Reciprocal(x="Sampling rate (Hz)") -> (1/x=w929:dbl)
    n640 = Multiply(x=w929, y=1000.0) -> (x*y=w927:dbl)
    n641 = Wait Until Next ms Multiple(millisecond multiple=w927) -> ()  [unwired: 1 out]
  }
  n642 = local read "Max Field (T)"() -> (w59:dbl)
  n643 = local read "Min Field (T)"() -> (w61:dbl)
  n644 = local read "dB (T)"() -> (w60:dbl)
  n645 = Divide(x=w59, y=w60) -> (x/y=w62:dbl)
  n646 = for {
    N: w62 -> [_]
    tunnel: w60 -> [w1283]
    tunnel: [w1280] -> w22 mode=indexing
    tunnel: w61 -> [w1281]
    tunnel: [0.0] -> _ mode=indexing
    i -> [w1284]
    n647 = Multiply(x=w1284, y=w1283) -> (x*y=w1282:dbl)
    n648 = Add(x=w1282, y=w1281) -> (x+y=w1280:dbl)
  }
  n649 = Multiply(x=w22, y=0.0) -> (x*y=w19:dbl[])
  n650 = Array Size(array=w19) -> (size(s)=w18:i32)
  n651 = Decrement(x=w18) -> (x-1=w17:i32)
  n652 = local write "B array"(w22) -> ()
  n653 = Array Subset(array=w19, length=w17) -> (w16:dbl[])  [unwired: 1 in]
  n654 = Build Array(w19, w19) -> (w20:dbl[][])
  n655 = local write "Averaged I(B)"(w20) -> ()
  n656 = Build Array(w16, w16) -> (w15:dbl[][])
  n657 = local write "Averaged P(B)"(w15) -> ()
  n658 = local write "Averaged dt"(w15) -> ()
  n659 = local read "Lake Shore"() -> (w72:refnum<visa-resource-name>)
  n660 = local read "IV converter"() -> (w88:refnum<visa-resource-name>)
  n661 = local read "Magnetic Field"() -> (w87:refnum<visa-resource-name>)
  n662 = VISA Close(VISA resource name=w88, error in (no error)=w90) -> (error out=w91:errorcluster)
  n663 = VISA Close(VISA resource name=w87, error in (no error)=w91) -> (error out=w89:errorcluster)
  n664 = Release Queue(queue=w97, error in (no error)=w89) -> (error out=w85:errorcluster)  [unwired: 1 in, 2 out]
  n665 = Merge Errors(w85, w84) -> (w86:errorcluster)
  n666 = VISA Close(VISA resource name=w72, error in (no error)=w86) -> (error out=w83:errorcluster)
  n667 = local read "refnum out"() -> (w81:refnum<file>)
  n668 = Close File(refnum=w81, error in=w83) -> (error out=w82:errorcluster)  [unwired: 1 out]
  n669 = call <vilib>:"Simple Error Handler.vi"("error in (no error)"=w82) -> ()  [unwired: 4 in, 5 out]
  "i" <- w52
  "j" <- w52
